vi "PowerRiderDLL_demo.vi"() -> ()   [LabVIEW 2017]
uses:
  Fuse25A_Labview/Power-Rider-GUI/CANalystII/PCAN_Driver/ControlCAN.llb/CAN Channel.ctl
  D:/Projects/GUI/Power Rider Wrapper/PowerRiderDLLWrapper.dll
  PowerRiderDLLWrapper.dll
  Fuse25A_Labview/Power-Rider-GUI/CANalystII/PCAN_Driver/ControlCAN.lvlib
panel:
  in  "TripType Enum":T1(ring)
  in  "Status Enum":enum16{"OFF", "ON", "ERROR", "FOREVER OFF"}(ring)
  out "ch_name":string
  out "unit_name":string
  out "sn_l":string
  out "PN ver":string
  out "SW ver":string
  in  "stop Int":bool
  out "RXdata":T2 {"ID" format="%.0x"}
  in  "Clear Dis":bool
  in  "stop m":bool
  out "String":string
  in  "Tab Control":T3(tab)
  in  "Send":bool
  in  "commandID":u32(ring)=33 items=["ChannelStatus_1"=0, "ChannelControl"=2, "Current_CH1_4"=3, "Current_CH5_8"=4, "Current_CH9_12"=5, "Current_CH13_16"=6, "GetVinVout"=8, "Version_BoardType"=9, "SystemTemp"=10, "SystemParameter"=11, "ChannelParameter"=12, "GetTripEvent"=15, "LogFile"=18, "Configuration"=19, "ProductionData"=20, "BIT"=33, "DiscretePorts"=34, "SerialNumber"=36, "OffsetMeasurement"=37, "PartNumber"=39, "ChannelCombinedStatus_1_CH1_8"=40, "ChannelCombinedStatus_2_CH9_12"=41, "PlotData"=45, "PlotCommand"=46, "InternalData"=47, "KeepAlive"=234, "WakeUp"=250]
  in  "systemParamNumber":u8(ring) items=["SystemUpTime", "UnitIDAddress", "R_Sense", "OpAmpGain", "RingCancelDelay", "VinLowThreshold", "VinHighThresholdP1", "TempLowThreshold", "TempHighThreshold", "GeneralString", "StatusMessage", "SysTime", "CAN_Bitrate", "SerialBaudrate", "DigOutDelayBeforeActive", "DigOutDelayBeforeDeactive", "DigOutOffTimeout", "DigOutControlLow", "DigOutLogicInverse", "DigInputType", "OutputStartupState", "PilotLED_FullScale", "UnitSubAddress", "DigOutControlHigh", "HostAddress", "LogFileDataTime", "OverVoltageTimeP1", "OverVoltageTimeP2", "OverVoltageTimeP3", "VinHighThresholdP2", "VinHighThresholdP3", "TotalUnitCurrentConsumptionScene1", "ChannelPrioritySceneNum", "InputFunctionMode", "InputLogicInverse", "TotalUnitCurrentConsumptionScene2", "TotalUnitCurrentConsumptionScene3", "OverVoltageVin1RetryDelay", "OverVoltageVin2RetryDelay", "VoltageLowHysteresis", "VoltageHighHysteresis", "CommunicationTimeout", "DigitalInputConfig"]
  in  "Sys Param":bool
  in  "CHParamNumber":u8(ring) items=["OverloadThreshold"=0, "Zone2Delay"=1, "HardShortRetryDelay"=2, "HardShortNumOfRetries"=3, "ActiveOnStartup"=4, "GeneralString"=5, "ChCommunicationControl"=6, "SW_TrippedRetryDelay"=7, "SW_TrippedNumOfRetries"=8, "ChStatusResetDelay"=9, "OverloadTime"=10, "I_MaxZone3Time"=11, "I_MaxZone3Threshold"=12, "NominalCurrentValue"=13, "I_2tThreshold"=14, "GroupChannelControl"=15, "TechData"=16, "PWM_Frequency"=17, "PWM_DutyCycle"=18, "PowerProtection"=19, "I_MaxZone2Threshold"=20, "PWM_Control"=21, "ChDelayBeforeOpening"=22, "ChDelayBeforeClosing"=23, "ChOffTimeout"=24, "LogicControl1"=25, "LogicControl2"=26, "I_MaxZone2Time"=27, "LogicControl3"=28, "LogicControl4"=29, "LogEventCurrentThreshold"=30, "OvervoltageNumOfRetries"=32, "ChannelPriorityScene1"=33, "ChannelPriorityScene2"=34, "ChannelPriorityScene3"=35, "I_MinThreshold"=36, "LossCommunicationChannelState"=37, "SoftStopPWM_DC"=38]
  in  "CH Param":bool
  in  "CH Cnt":bool
  in  "SW reset":bool
  in  "Get PN":bool
  in  "Get SW ver":bool
  in  "Get CH Current":bool
  in  "Get CH STS":bool
  in  "Get CH Voltage":bool
  in  "Get CH Name":bool
  in  "Get SN":bool
  in  "Get Unit Name":bool
  in  "Com type":enum32{"CAN", "Serial", "UDP"}(tab)
  in  "Baud":u32(ring)=250000 items=["1M"=1000000, "800K"=800000, "500K"=500000, "250K"=250000, "125K"=125000, "100K"=100000, "83.3K"=83300, "50000"=50000, "20K"=20000, "10K"=10000, "5K"=5000]
  in  "Channel #":T4 caption="Channel" items=["Channel 1", "Channel 2"]
  in  "VISA res_in":refnum<visa-resource-name>
  in  "baud rate":u32(ring)=19200 items=["921600"=921600, "460800"=460800, "256000"=256000, "115200"=115200, "57600"=57600, "38400"=38400, "19200"=19200, "14400"=14400, "9600"=9600, "2400"=2400, "1200"=1200]
  in  "address IP":string="192.168.1.50"
  in  "Port":u16=8030
  in  "Select CH #":u8(ring)=1 items=["CH1"=1, "CH2"=2, "CH3"=3, "CH4"=4, "CH5"=5, "CH6"=6, "CH7"=7, "CH8"=8, "CH9"=9, "CH10"=10, "CH11"=11, "CH12"=12, "CH13"=13, "CH14"=14, "CH15"=15, "CH16"=16]
  out "SendOK":bool
  out "path":path
  out "COM":variant
  out "PowerAddress":u8
  out "HostAddress":u8
  out "CommandID":u8 format="%.0x"
  in  "Dst add":u16=16 format="%.0x"
  in  "address":u16=85 format="%.0x"
  in  "Disonnect":bool
  in  "Connect":bool
  out "CommIcon":bool
  in  "COMType":u16(ring)=2 items=["CANalystII"=2, "TCP Client"=3, "TCP Server"=4, "UDP Client"=5, "Serial COM"=6, "CAN Kvaser"=7]
  in  "payload":u8[](array[numeric])
  out "Payload":u8[](array[numeric]) format="%.0x"
  # "Communication"
  # "Commands"
  # "Responds"
  # "ver 0.1.a"
  # "Power Rider"
  # "REDLER TECHNOLOGIES LTD"
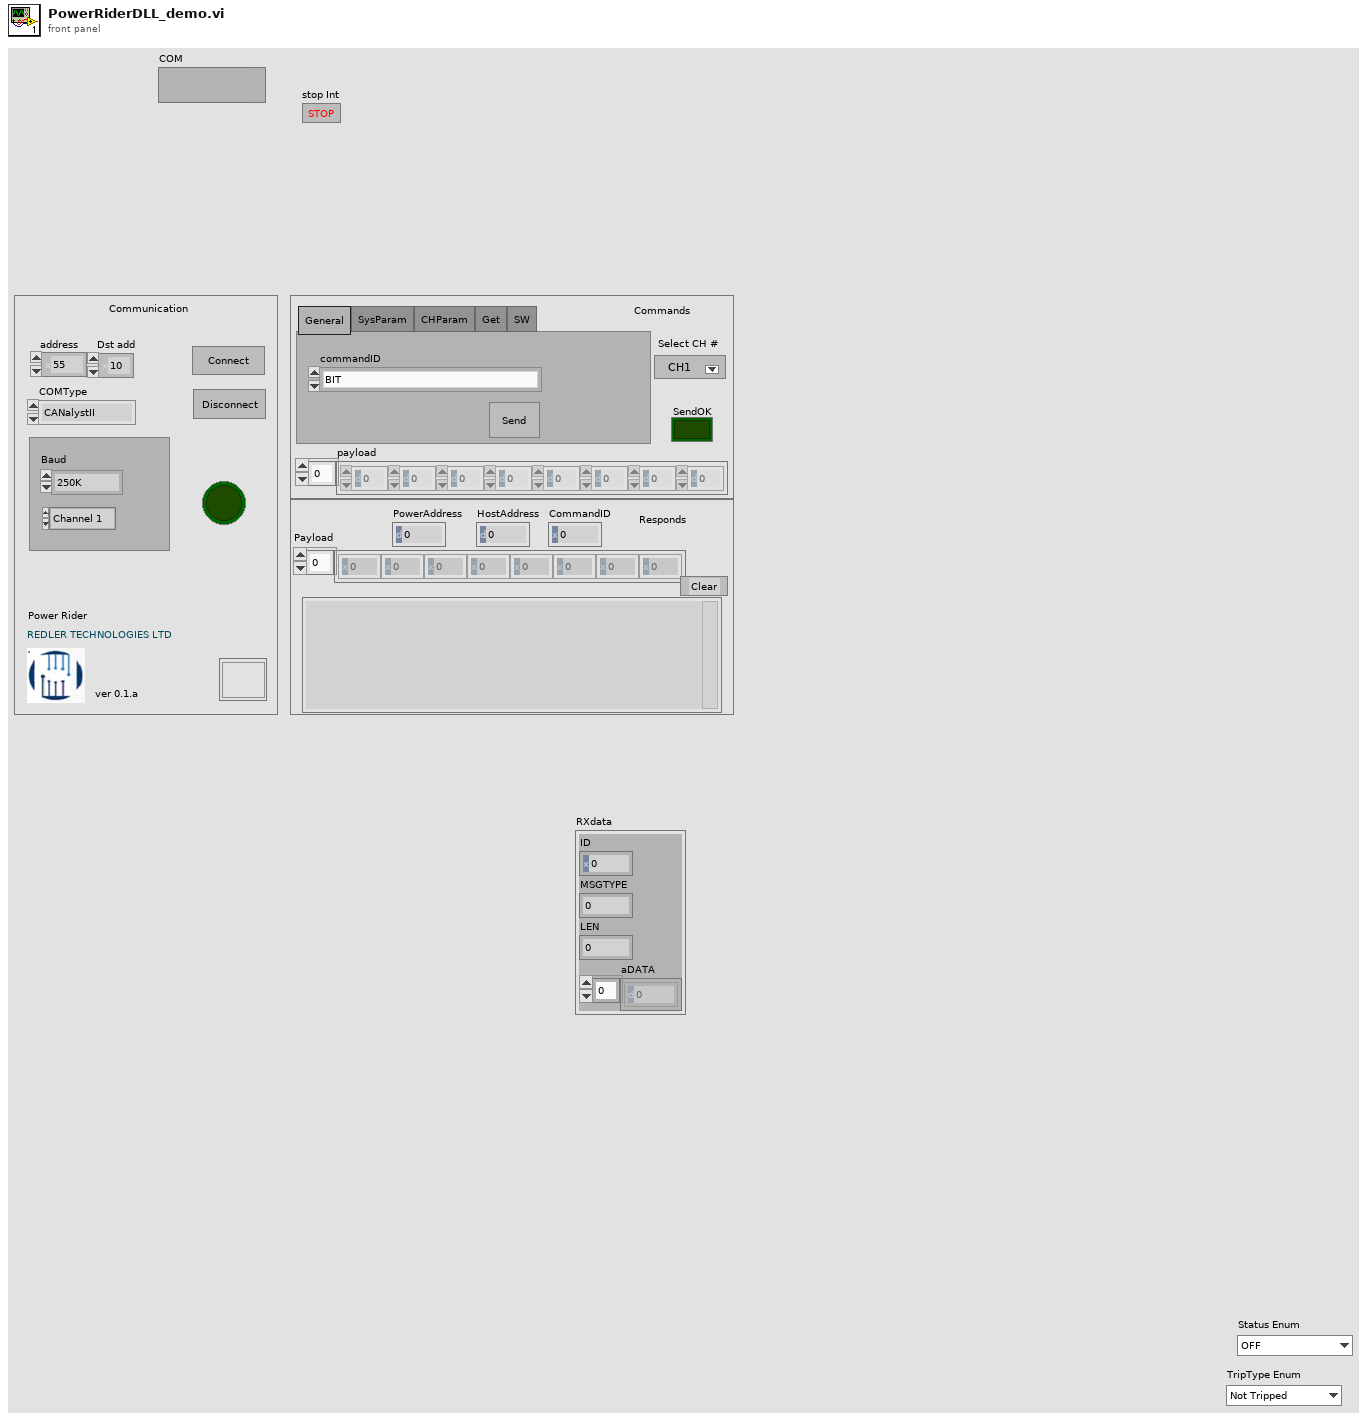
[diagram p1: front panel]
types:
  T1 = enum16{"Not Tripped", "SW Tripped", "Hard Short", "MAX SW Tripped"}
  T2 = cluster{"ID":u32, "MSGTYPE":u8, "LEN":u8, "aDATA":u8[]}
  T3 = enum32{"General", "SysParam", "CHParam", "Get", "SW"}
  T4 = typedef "ControlCAN.lvlib/CAN Channel.ctl" = u32
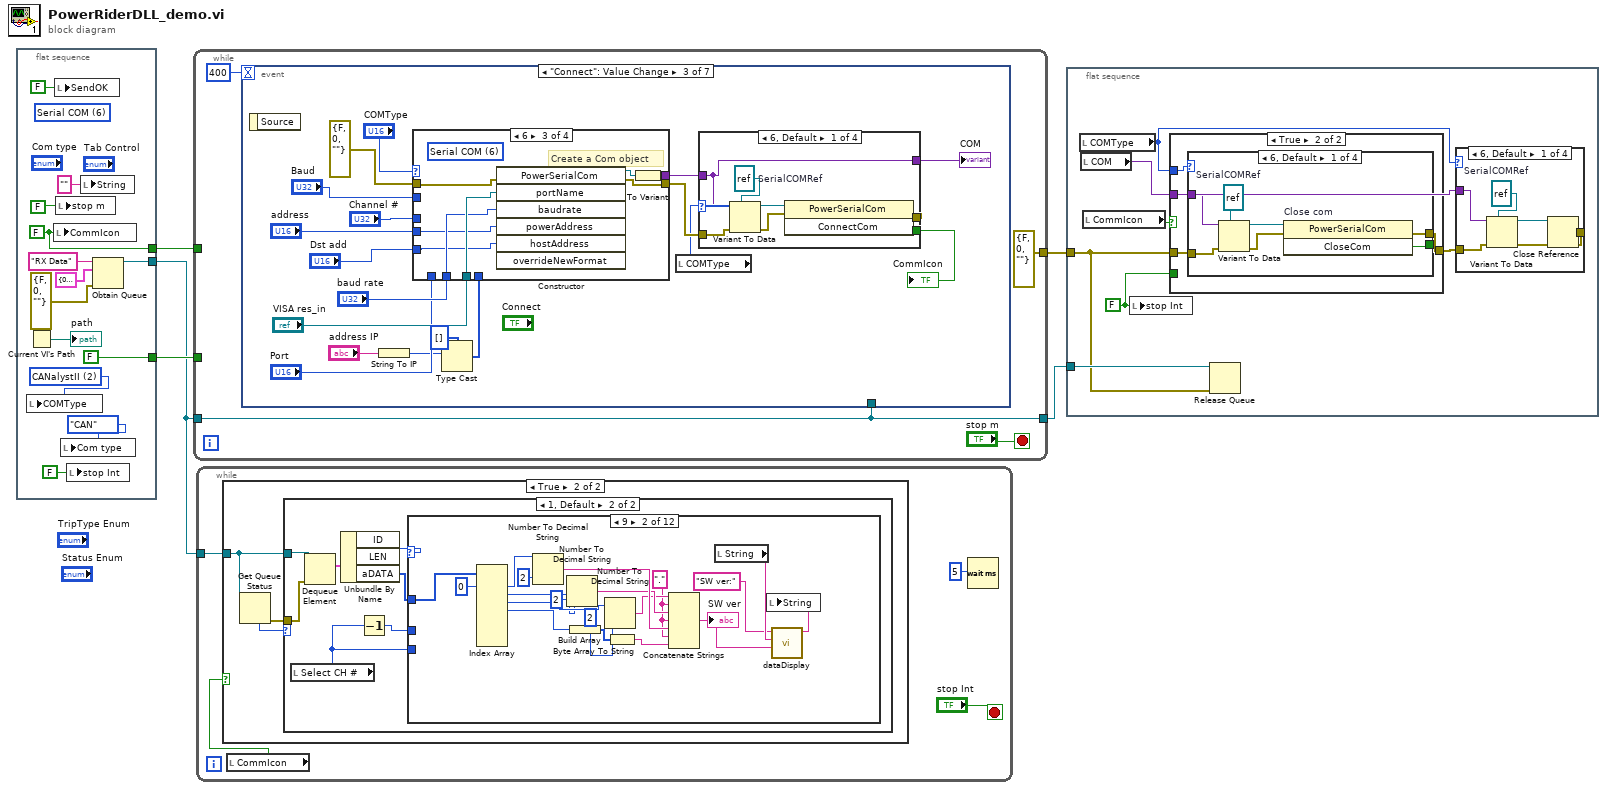
[diagram p0: block diagram]
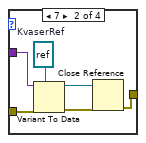
[diagram p2: hidden frame]
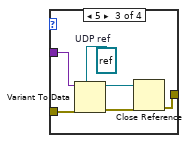
[diagram p3: hidden frame]
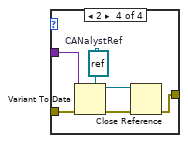
[diagram p4: hidden frame]
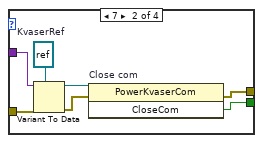
[diagram p6: hidden frame]
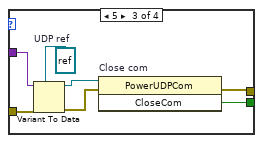
[diagram p7: hidden frame]
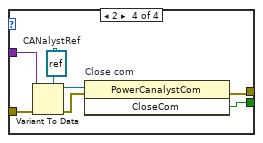
[diagram p8: hidden frame]
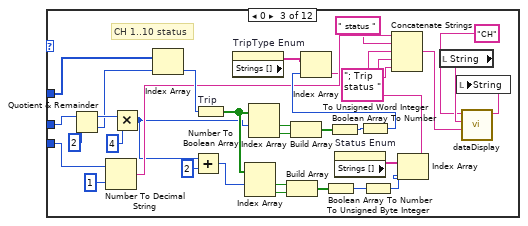
[diagram p12: hidden frame]
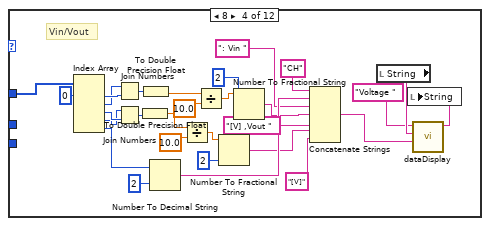
[diagram p13: hidden frame]
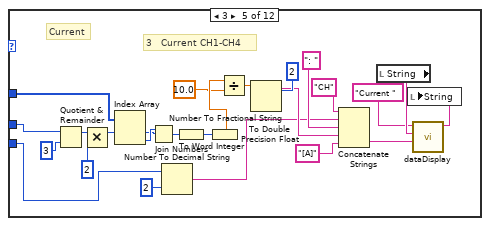
[diagram p14: hidden frame]
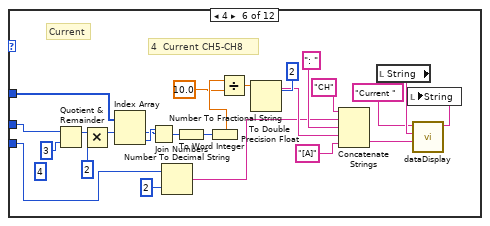
[diagram p15: hidden frame]
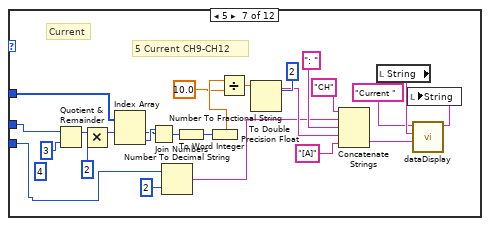
[diagram p16: hidden frame]
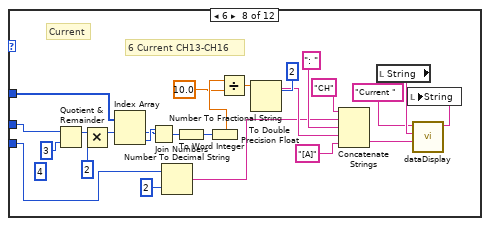
[diagram p17: hidden frame]
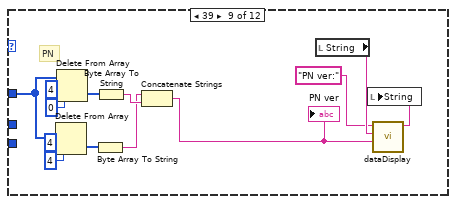
[diagram p18: hidden frame]
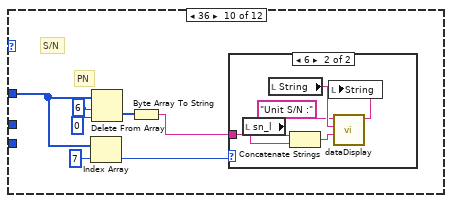
[diagram p19: hidden frame]
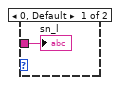
[diagram p20: hidden frame]
diagram:
  n1 = flat-sequence {
    tunnel: [FALSE] -> w4
    tunnel: [w14] -> w3
    tunnel: [w7] -> w2
    frame #0 {
      (unwired) u16 6 items=["CANalystII"=2, "TCP Client"=3, "TCP Server"=4, "UDP Client"=5, "Serial COM"=6, "CAN Kvaser"=7] ("COMType 2")
      w14 = FALSE ("CommIcon")
      w16 = u16 2 items=["CANalystII"=2, "TCP Client"=3, "TCP Server"=4, "UDP Client"=5, "Serial COM"=6, "CAN Kvaser"=7] ("COMType")
      n2 = Current VI's Path() -> (path=→"path":path)
      n3 = local write "COMType"(w16) -> ()
      n4 = local write "CommIcon"(w14) -> ()
      n5 = local write "SendOK"(FALSE ("SendOK")) -> ()
      n6 = local write "stop m"(FALSE ("Exit")) -> ()
      n7 = local write "Com type"(enum32{"CAN", "Serial", "UDP"}."CAN" ("Com type")) -> ()
      n8 = local write "stop Int"(FALSE ("stop Int")) -> ()
      n9 = local write "String"("" ("String")) -> ()
      n10 = Obtain Queue(name (unnamed)="RX Data", element data type=T2 {"ID"=0, "MSGTYPE"=0, "LEN"=0, "aDATA"=[]} ("Msg"), error in (no error)=errorcluster {"status"=FALSE, "code"=0, "source"=""}) -> (queue out=w7:refnum<queue>)  [unwired: 2 in, 2 out]
    }
  }
  n11 = while {
    tunnel: [errorcluster {"status"=FALSE, "code"=0, "source"=""} ("error out")] -> w5
    tunnel: w4 -> [_]
    tunnel: w3 -> [_]
    tunnel: w2 -> [w19]
    tunnel: [w19] -> w1
    stop <- "stop m" stop-if-true
    n12 = event shown="[2] \"Connect\": Value Change" {
      selector: _ -> [_ _ _ _ _ _ _]
      dyn-events: _ -> [_ _ _ _ _ _ _]
      timeout: 400 -> [_ _ _ _ _ _ _]
      tunnel: w19 -> [w23 _ _ _ _ _ _]
      event Timeout {
        n13 = event-data() -> ()  [unwired: 1 in, 1 out]
        n14 = local read "CommIcon"() -> (w24:bool)
        n15 = case shown="True" w24 {
          tunnel: w23 -> [_ w31]
          frame False {
          }
          frame True {
            n16 = local read "COM"() -> (w34:variant)
            n17 = local read "COMType"() -> (w32:u16)
            n18 = case shown="6" w32 {
              selector: w32 -> [w61 w70 w95 w97]
              tunnel: w34 -> [w68 w82 w85 w109]
              tunnel: errorcluster {"status"=FALSE, "code"=0, "source"=""} ("error out") -> [w66 w81 w84 w108]
              tunnel: [w56 w75 w92 w102] -> w29
              tunnel: [w57 w74 w91 w101] -> w30
              tunnel: [w58 w73 w90 w100] -> w28
              tunnel: [w59 w72 w89 w99] -> w27
              tunnel: [w60 w71 w88 w98] -> w26
              tunnel: [w61 w70 w95 w97] -> w25
              tunnel: [w55 w69 w83 w96] -> _
              frame 2, Default {
                w67 = refnum<k24> refnum  # CANalystRef
                n19 = Variant To Data(error in=w66, type=w67, Variant=w68) -> (data=w65:refnum<k24>, error out=w64:errorcluster)
                n20 = invoke class="PowerCanalystCom" method="ReceivePacket"(reference=w65, error in=w64) -> (error out=w62:errorcluster, "ReceivePacket"=w63:refnum<k24>)  [unwired: 1 in, 1 out]
                n21 = property class="PowerPacket"(reference=w63, error in=w62) -> (error out=w55:errorcluster, "CommandID"=w56:u8, "ErrorFlag"=w57:bool, "HostAddress"=w58:u8, "PowerAddress"=w59:u8, "MutablePayload"=w60:u8[])  [unwired: 1 out]
              }
              frame 6 {
                w76 = refnum<k24> refnum  # SerialCOMRef
                n22 = Variant To Data(error in=w81, type=w76, Variant=w82) -> (data=w80:refnum<k24>, error out=w79:errorcluster)
                n23 = invoke class="PowerSerialCom" method="ReceivePacket"(reference=w80, error in=w79) -> (error out=w77:errorcluster, "ReceivePacket"=w78:refnum<k24>)  [unwired: 1 in, 1 out]
                n24 = property class="PowerPacket"(reference=w78, error in=w77) -> (error out=w69:errorcluster, "CommandID"=w75:u8, "ErrorFlag"=w74:bool, "HostAddress"=w73:u8, "PowerAddress"=w72:u8, "MutablePayload"=w71:u8[])  [unwired: 1 out]
              }
              frame 5 {
                w87 = refnum<k24> refnum  # UDP ref
                n25 = Variant To Data(error in=w84, type=w87, Variant=w85) -> (data=w86:refnum<k24>)  [unwired: 1 out]
                n26 = invoke class="PowerUDPCom" method="ReceivePacketAsync"(reference=w86) -> ("ReceivePacketAsync"=w94:refnum<k24>)  [unwired: 2 in, 2 out]
                n27 = property class="Task`1[[PowerRiderDLLWrapper.Po"(reference=w94) -> ("Result"=w93:refnum<k24>)  [unwired: 1 in, 2 out]
                n28 = property class="PowerPacket"(reference=w93) -> (error out=w83:errorcluster, "CommandID"=w92:u8, "ErrorFlag"=w91:bool, "HostAddress"=w90:u8, "PowerAddress"=w89:u8, "MutablePayload"=w88:u8[])  [unwired: 1 in, 1 out]
              }
              frame 7 {
                w103 = refnum<k24> refnum  # KvaserRef
                n29 = Variant To Data(error in=w108, type=w103, Variant=w109) -> (data=w107:refnum<k24>, error out=w106:errorcluster)
                n30 = invoke class="PowerKvaserCom" method="ReceivePacket"(reference=w107, error in=w106) -> (error out=w104:errorcluster, "ReceivePacket"=w105:refnum<k24>)  [unwired: 1 in, 1 out]
                n31 = property class="PowerPacket"(reference=w105, error in=w104) -> (error out=w96:errorcluster, "CommandID"=w102:u8, "ErrorFlag"=w101:bool, "HostAddress"=w100:u8, "PowerAddress"=w99:u8, "MutablePayload"=w98:u8[])  [unwired: 1 out]
              }
            }
            n32 = case shown="False" w30 {
              tunnel: w26 -> [w39 w47]
              tunnel: w27 -> [w45 _]
              tunnel: w28 -> [w46 _]
              tunnel: w29 -> [w40 _]
              tunnel: w25 -> [w38 _]
              tunnel: w31 -> [w36 _]
              frame False {
                # "OK"
                n33 = local read "String"() -> (w43:string)
                n34 = call "StrDisplay.vi"("Payload"=w39, "ID"=w40, "string in"=w43, "string type"="RX") -> ("str out"=→"String":string)  [unwired: 7 in]
                n35 = Bundle By Name(cluster=T2 {"ID"=0, "MSGTYPE"=0, "LEN"=0, "aDATA"=[]} ("Msg"), "ID"=w40, "MSGTYPE"=w38, "LEN"=u8 0, "aDATA"=w39) -> (w35:T2)
                "RXdata" <- w35
                n36 = Enqueue Element(queue=w36, element=w35) -> ()  [unwired: 1 in, 4 out]
                "Payload" <- w39
                "CommandID" <- w40
                "HostAddress" <- w46
                "PowerAddress" <- w45
              }
              frame True {
                n37 = Index Array(array=w47, index=0) -> (element=w48:u8)
                n38 = case shown="1, Default" w48 {
                  tunnel: w48 -> [_ w54]
                  tunnel: w47 -> [_ _]
                  frame 9 {
                  }
                  frame 1, Default {
                    # "Error"
                    n39 = Number To Decimal String(number=w54) -> (decimal integer string=w50:string)  [unwired: 1 in]
                    n40 = local read "String"() -> (w52:string)
                    n41 = call "StrDisplay.vi"("Err str"=w50, "string in"=w52, "string type"="Error") -> ("str out"=w53:string)  [unwired: 8 in]
                    n42 = local write "String"(w53) -> ()
                  }
                }
              }
            }
          }
        }
      }
      event "Clear Dis": Value Change {
        n43 = event-data() -> ()  [unwired: 1 in, 6 out]
        n44 = local write "String"("" ("String")) -> ()
      }
      event "Connect": Value Change {
        n45 = event-data() -> ()  [unwired: 1 in, 1 out]
        n46 = String To IP(1:"address IP") -> (0:w113:u32)
        n47 = Type Cast(type=u8[] [] ("powerIPAddress"), x=w113) -> (*(type *) &x=w111:u8[])
        n48 = case shown="6" "COMType" {
          tunnel: [w164 w172 w180 w188] -> w125
          tunnel: [w157 w166 w178 w186] -> w126
          tunnel: "Baud" -> [w162 w170 _ _]
          tunnel: "Dst add" -> [w159 w167 w173 w181]
          tunnel: "address" -> [w160 w168 w174 w182]
          tunnel: "Channel #" -> [w161 w169 _ _]
          tunnel: errorcluster {"status"=FALSE, "code"=0, "source"=""} ("error out") -> [w163 w171 w177 w185]
          tunnel: "baud rate" -> [_ _ w175 _]
          tunnel: "VISA res_in" -> [_ _ w176 _]
          tunnel: "Port" -> [_ _ _ w183]
          tunnel: w111 -> [_ _ _ w184]
          frame 2, Default {
            (unwired) u16 2 items=["CANalystII"=2, "TCP Client"=3, "TCP Server"=4, "UDP Client"=5, "Serial COM"=6, "CAN Kvaser"=7] ("COMType 2")
            n49 = constructor class="PowerCanalystCom"(error in=w163, "bitrate"=w162, "deviceIndex"=w161, "powerAddress"=w160, "hostAddress"=w159) -> (reference out=w158:refnum<k24>, error out=w157:errorcluster)  [unwired: 2 in, 5 out]
            n50 = To Variant(anything=w158) -> (Variant=w164:variant)
          }
          frame 7 {
            (unwired) u16 7 items=["CANalystII"=2, "TCP Client"=3, "TCP Server"=4, "UDP Client"=5, "Serial COM"=6, "CAN Kvaser"=7] ("COMType 2")
            n51 = constructor class="PowerKvaserCom"(error in=w171, "bitrate"=w170, "deviceIndex"=w169, "powerAddress"=w168, "hostAddress"=w167) -> (reference out=w165:refnum<k24>, error out=w166:errorcluster)  [unwired: 2 in, 5 out]
            n52 = To Variant(anything=w165) -> (Variant=w172:variant)
          }
          frame 6 {
            (unwired) u16 6 items=["CANalystII"=2, "TCP Client"=3, "TCP Server"=4, "UDP Client"=5, "Serial COM"=6, "CAN Kvaser"=7] ("COMType 2")
            # "Create a Com object"
            n53 = constructor class="PowerSerialCom"(error in=w177, "portName"=w176, "baudrate"=w175, "powerAddress"=w174, "hostAddress"=w173) -> (reference out=w179:refnum<k24>, error out=w178:errorcluster)  [unwired: 3 in, 6 out]
            n54 = To Variant(anything=w179) -> (Variant=w180:variant)
          }
          frame 5 {
            (unwired) u16 5 items=["CANalystII"=2, "TCP Client"=3, "TCP Server"=4, "UDP Client"=5, "Serial COM"=6, "CAN Kvaser"=7] ("COMType 2")
            n55 = constructor class="PowerUDPCom"(error in=w185, "powerIPAddress"=w184, "powerPort"=w183, "powerAddress"=w182, "hostAddress"=w181) -> (reference out=w187:refnum<k24>, error out=w186:errorcluster)  [unwired: 2 in, 5 out]
            n56 = To Variant(anything=w187) -> (Variant=w188:variant)
          }
        }
        n57 = local read "COMType"() -> (w124:u16)
        n58 = case shown="6, Default" w124 {
          tunnel: w125 -> [w129 w136 w143 w151]
          tunnel: [w131 w137 w146 w154] -> w128
          tunnel: w126 -> [w135 w142 w145 w153]
          tunnel: [w130 w138 w144 w152] -> _
          tunnel: [w129 w136 w143 w151] -> w116
          frame 6, Default {
            w134 = refnum<k24> refnum  # SerialCOMRef
            n59 = Variant To Data(error in=w135, type=w134, Variant=w129) -> (data=w133:refnum<k24>, error out=w132:errorcluster)
            n60 = invoke class="PowerSerialCom" method="ConnectCom"(reference=w133, error in=w132) -> (error out=w130:errorcluster, "ConnectCom"=w131:bool)  [unwired: 1 in, 1 out]
          }
          frame 7 {
            w139 = refnum<k24> refnum  # KvaserRef
            n61 = Variant To Data(error in=w142, type=w139, Variant=w136) -> (data=w140:refnum<k24>, error out=w141:errorcluster)
            n62 = invoke class="PowerKvaserCom" method="ConnectCom"(reference=w140, error in=w141) -> (error out=w138:errorcluster, "ConnectCom"=w137:bool)  [unwired: 1 in, 1 out]
          }
          frame 2 {
            w149 = refnum<k24> refnum  # CANalystRef
            n63 = Variant To Data(error in=w145, type=w149, Variant=w143) -> (data=w148:refnum<k24>, error out=w147:errorcluster)
            n64 = invoke class="PowerCanalystCom" method="ConnectCom"(reference=w148, error in=w147) -> (error out=w144:errorcluster, "ConnectCom"=w146:bool)  [unwired: 1 in, 1 out]
          }
          frame 5 {
            w150 = refnum<k24> refnum  # UDP ref
            n65 = Variant To Data(error in=w153, type=w150, Variant=w151) -> (data=w156:refnum<k24>, error out=w155:errorcluster)
            n66 = invoke class="PowerUDPCom" method="ConnectCom"(reference=w156, error in=w155) -> (error out=w152:errorcluster, "ConnectCom"=w154:bool)  [unwired: 1 in, 1 out]
          }
        }
        "CommIcon" <- w128
        "COM" <- w116
      }
      event "Get SW ver", "Get CH Voltage", "Get CH STS", "Get CH Current", "Get PN", "SW reset", "Get SN", "Get CH Name", "Get Unit Name", "CH Cnt": Value Change {
        w189 = FALSE ("SendOK")
        n67 = event-data() -> ("CtlRef"=w192:refnum<vi>)  [unwired: 1 in]
        n68 = local write "SendOK"(w189) -> ()
        n69 = local read "CommIcon"() -> (w198:bool)
        n70 = property class="Bool"(reference=w192) -> ("Label.Text"=w191:string)  [unwired: 1 in, 2 out]
        n71 = local read "COM"() -> (w199:variant)
        n72 = local read "COMType"() -> (w200:u16)
        n73 = case shown="True" w198 {
          tunnel: w200 -> [_ w210]
          tunnel: u8 6 ("priority") -> [_ w209]
          tunnel: "commandID" -> [_ w208]
          tunnel: "payload" -> [_ w207]
          tunnel: w199 -> [_ w206]
          tunnel: errorcluster {"status"=FALSE, "code"=0, "source"=""} ("error out") -> [_ w205]
          tunnel: [FALSE ("SendPacket") w204] -> w193
          tunnel: w191 -> [_ w203]
          tunnel: "Select CH #" -> [_ w202]
          tunnel: w189 -> [_ _]
          frame False {
          }
          frame True {
            n74 = case shown="6, Default" w210 {
              tunnel: w206 -> [w222 w350 w478 w606]
              tunnel: [w211 w339 w473 w601] -> w204
              tunnel: w205 -> [w221 w349 w476 w605]
              tunnel: [w212 w347 w474 w602] -> _
              tunnel: w209 -> [w216 w343 w471 w600]
              tunnel: w208 -> [w215 w342 w470 w599]
              tunnel: w207 -> [w214 w341 w469 w598]
              tunnel: w203 -> [w219 w346 w467 w603]
              tunnel: w202 -> [w213 w340 w468 w597]
              frame 6, Default {
                w220 = refnum<k24> refnum  # SerialCOMRef
                n75 = Variant To Data(error in=w221, type=w220, Variant=w222) -> (data=w217:refnum<k24>, error out=w218:errorcluster)
                n76 = case shown="\"Get SW ver\"" w219 {
                  tunnel: w218 -> [w229 w236 w243 w250 w257 w265 w277 w303 w306 w312 w317 w329 w336]
                  tunnel: [w228 w235 w242 w249 w256 w264 w276 w302 w308 w315 w321 w332 w335] -> w212
                  tunnel: [w227 w234 w241 w248 w255 w263 w275 w301 w309 w314 w324 w331 w334] -> w211
                  tunnel: w217 -> [w226 w233 w240 w247 w254 w262 w274 w300 w307 w313 w318 w330 w337]
                  tunnel: w216 -> [w225 w232 w239 w246 w253 w261 w273 w299 w305 w311 w323 w328 w338]
                  tunnel: w215 -> [w224 _ _ _ _ _ _ _ _ _ _ _ _]
                  tunnel: w214 -> [w223 w231 w238 w245 w252 w260 _ _ _ _ w320 w326 _]
                  tunnel: w213 -> [_ _ _ _ _ w258 w271 w287 _ _ w322 _ w333]
                  frame "Send", Default {
                    n77 = invoke class="PowerSerialCom" method="SendPacket"(reference=w226, error in=w229, "priority"=w225, "commandID"=w224, "payload"=w223) -> (error out=w228:errorcluster, "SendPacket"=w227:bool)  [unwired: 1 in, 4 out]
                  }
                  frame "Get SW ver" {
                    w230 = u8 9 items=["ChannelStatus_1"=0, "ChannelControl"=2, "Current_CH1_4"=3, "Current_CH5_8"=4, "Current_CH9_12"=5, "Current_CH13_16"=6, "GetVinVout"=8, "Version_BoardType"=9, "SystemTemp"=10, "SystemParameter"=11, "ChannelParameter"=12, "GetTripEvent"=15, "LogFile"=18, "Configuration"=19, "ProductionData"=20, "BIT"=33, "DiscretePorts"=34, "SerialNumber"=36, "OffsetMeasurement"=37, "PartNumber"=39, "ChannelCombinedStatus_1_CH1_8"=40, "ChannelCombinedStatus_2_CH9_12"=41, "PlotData"=45, "PlotCommand"=46, "InternalData"=47, "KeepAlive"=234, "WakeUp"=250] ("commandID")
                    n78 = invoke class="PowerSerialCom" method="SendPacket"(reference=w233, error in=w236, "priority"=w232, "commandID"=w230, "payload"=w231) -> (error out=w235:errorcluster, "SendPacket"=w234:bool)  [unwired: 1 in, 4 out]
                  }
                  frame "Get PN" {
                    w237 = u8 39 items=["ChannelStatus_1"=0, "ChannelControl"=2, "Current_CH1_4"=3, "Current_CH5_8"=4, "Current_CH9_12"=5, "Current_CH13_16"=6, "GetVinVout"=8, "Version_BoardType"=9, "SystemTemp"=10, "SystemParameter"=11, "ChannelParameter"=12, "GetTripEvent"=15, "LogFile"=18, "Configuration"=19, "ProductionData"=20, "BIT"=33, "DiscretePorts"=34, "SerialNumber"=36, "OffsetMeasurement"=37, "PartNumber"=39, "ChannelCombinedStatus_1_CH1_8"=40, "ChannelCombinedStatus_2_CH9_12"=41, "PlotData"=45, "PlotCommand"=46, "InternalData"=47, "KeepAlive"=234, "WakeUp"=250] ("commandID")
                    n79 = invoke class="PowerSerialCom" method="SendPacket"(reference=w240, error in=w243, "priority"=w239, "commandID"=w237, "payload"=w238) -> (error out=w242:errorcluster, "SendPacket"=w241:bool)  [unwired: 1 in, 4 out]
                  }
                  frame "SW reset" {
                    w244 = u8 36 items=["ChannelStatus_1"=0, "ChannelControl"=2, "Current_CH1_4"=3, "Current_CH5_8"=4, "Current_CH9_12"=5, "Current_CH13_16"=6, "GetVinVout"=8, "Version_BoardType"=9, "SystemTemp"=10, "SystemParameter"=11, "ChannelParameter"=12, "GetTripEvent"=15, "LogFile"=18, "Configuration"=19, "ProductionData"=20, "BIT"=33, "DiscretePorts"=34, "SerialNumber"=36, "OffsetMeasurement"=37, "PartNumber"=39, "ChannelCombinedStatus_1_CH1_8"=40, "ChannelCombinedStatus_2_CH9_12"=41, "PlotData"=45, "PlotCommand"=46, "InternalData"=47, "KeepAlive"=234, "WakeUp"=250] ("commandID")
                    n80 = invoke class="PowerSerialCom" method="SendPacket"(reference=w247, error in=w250, "priority"=w246, "commandID"=w244, "payload"=w245) -> (error out=w249:errorcluster, "SendPacket"=w248:bool)  [unwired: 1 in, 4 out]
                  }
                  frame "Get CH STS" {
                    w251 = u8 0 items=["ChannelStatus_1"=0, "ChannelControl"=2, "Current_CH1_4"=3, "Current_CH5_8"=4, "Current_CH9_12"=5, "Current_CH13_16"=6, "GetVinVout"=8, "Version_BoardType"=9, "SystemTemp"=10, "SystemParameter"=11, "ChannelParameter"=12, "GetTripEvent"=15, "LogFile"=18, "Configuration"=19, "ProductionData"=20, "BIT"=33, "DiscretePorts"=34, "SerialNumber"=36, "OffsetMeasurement"=37, "PartNumber"=39, "ChannelCombinedStatus_1_CH1_8"=40, "ChannelCombinedStatus_2_CH9_12"=41, "PlotData"=45, "PlotCommand"=46, "InternalData"=47, "KeepAlive"=234, "WakeUp"=250] ("commandID")
                    n81 = invoke class="PowerSerialCom" method="SendPacket"(reference=w254, error in=w257, "priority"=w253, "commandID"=w251, "payload"=w252) -> (error out=w256:errorcluster, "SendPacket"=w255:bool)  [unwired: 1 in, 4 out]
                  }
                  frame "Get CH Current" {
                    n82 = case shown="1..4, Default" w258 {
                      tunnel: [w266 w267 w268 w269] -> w259
                      frame 1..4, Default {
                        w266 = u8 3 items=["ChannelStatus_1"=0, "ChannelControl"=2, "Current_CH1_4"=3, "Current_CH5_8"=4, "Current_CH9_12"=5, "Current_CH13_16"=6, "GetVinVout"=8, "Version_BoardType"=9, "SystemTemp"=10, "SystemParameter"=11, "ChannelParameter"=12, "GetTripEvent"=15, "LogFile"=18, "Configuration"=19, "ProductionData"=20, "BIT"=33, "DiscretePorts"=34, "SerialNumber"=36, "OffsetMeasurement"=37, "PartNumber"=39, "ChannelCombinedStatus_1_CH1_8"=40, "ChannelCombinedStatus_2_CH9_12"=41, "PlotData"=45, "PlotCommand"=46, "InternalData"=47, "KeepAlive"=234, "WakeUp"=250] ("commandID")
                      }
                      frame 5..8 {
                        w267 = u8 4 items=["ChannelStatus_1"=0, "ChannelControl"=2, "Current_CH1_4"=3, "Current_CH5_8"=4, "Current_CH9_12"=5, "Current_CH13_16"=6, "GetVinVout"=8, "Version_BoardType"=9, "SystemTemp"=10, "SystemParameter"=11, "ChannelParameter"=12, "GetTripEvent"=15, "LogFile"=18, "Configuration"=19, "ProductionData"=20, "BIT"=33, "DiscretePorts"=34, "SerialNumber"=36, "OffsetMeasurement"=37, "PartNumber"=39, "ChannelCombinedStatus_1_CH1_8"=40, "ChannelCombinedStatus_2_CH9_12"=41, "PlotData"=45, "PlotCommand"=46, "InternalData"=47, "KeepAlive"=234, "WakeUp"=250] ("commandID")
                      }
                      frame 9..12 {
                        w268 = u8 5 items=["ChannelStatus_1"=0, "ChannelControl"=2, "Current_CH1_4"=3, "Current_CH5_8"=4, "Current_CH9_12"=5, "Current_CH13_16"=6, "GetVinVout"=8, "Version_BoardType"=9, "SystemTemp"=10, "SystemParameter"=11, "ChannelParameter"=12, "GetTripEvent"=15, "LogFile"=18, "Configuration"=19, "ProductionData"=20, "BIT"=33, "DiscretePorts"=34, "SerialNumber"=36, "OffsetMeasurement"=37, "PartNumber"=39, "ChannelCombinedStatus_1_CH1_8"=40, "ChannelCombinedStatus_2_CH9_12"=41, "PlotData"=45, "PlotCommand"=46, "InternalData"=47, "KeepAlive"=234, "WakeUp"=250] ("commandID")
                      }
                      frame 13..16 {
                        w269 = u8 6 items=["ChannelStatus_1"=0, "ChannelControl"=2, "Current_CH1_4"=3, "Current_CH5_8"=4, "Current_CH9_12"=5, "Current_CH13_16"=6, "GetVinVout"=8, "Version_BoardType"=9, "SystemTemp"=10, "SystemParameter"=11, "ChannelParameter"=12, "GetTripEvent"=15, "LogFile"=18, "Configuration"=19, "ProductionData"=20, "BIT"=33, "DiscretePorts"=34, "SerialNumber"=36, "OffsetMeasurement"=37, "PartNumber"=39, "ChannelCombinedStatus_1_CH1_8"=40, "ChannelCombinedStatus_2_CH9_12"=41, "PlotData"=45, "PlotCommand"=46, "InternalData"=47, "KeepAlive"=234, "WakeUp"=250] ("commandID")
                      }
                    }
                    n83 = invoke class="PowerSerialCom" method="SendPacket"(reference=w262, error in=w265, "priority"=w261, "commandID"=w259, "payload"=w260) -> (error out=w264:errorcluster, "SendPacket"=w263:bool)  [unwired: 1 in, 4 out]
                  }
                  frame "Get CH Voltage" {
                    w272 = u8 8 items=["ChannelStatus_1"=0, "ChannelControl"=2, "Current_CH1_4"=3, "Current_CH5_8"=4, "Current_CH9_12"=5, "Current_CH13_16"=6, "GetVinVout"=8, "Version_BoardType"=9, "SystemTemp"=10, "SystemParameter"=11, "ChannelParameter"=12, "GetTripEvent"=15, "LogFile"=18, "Configuration"=19, "ProductionData"=20, "BIT"=33, "DiscretePorts"=34, "SerialNumber"=36, "OffsetMeasurement"=37, "PartNumber"=39, "ChannelCombinedStatus_1_CH1_8"=40, "ChannelCombinedStatus_2_CH9_12"=41, "PlotData"=45, "PlotCommand"=46, "InternalData"=47, "KeepAlive"=234, "WakeUp"=250] ("commandID")
                    n84 = Build Array(w271) -> (w270:u8[])
                    n85 = invoke class="PowerSerialCom" method="SendPacket"(reference=w274, error in=w277, "priority"=w273, "commandID"=w272, "payload"=w270) -> (error out=w276:errorcluster, "SendPacket"=w275:bool)  [unwired: 1 in, 4 out]
                  }
                  frame "CH Cnt" {
                    w298 = u8 2 items=["ChannelStatus_1"=0, "ChannelControl"=2, "Current_CH1_4"=3, "Current_CH5_8"=4, "Current_CH9_12"=5, "Current_CH13_16"=6, "GetVinVout"=8, "Version_BoardType"=9, "SystemTemp"=10, "SystemParameter"=11, "ChannelParameter"=12, "GetTripEvent"=15, "LogFile"=18, "Configuration"=19, "ProductionData"=20, "BIT"=33, "DiscretePorts"=34, "SerialNumber"=36, "OffsetMeasurement"=37, "PartNumber"=39, "ChannelCombinedStatus_1_CH1_8"=40, "ChannelCombinedStatus_2_CH9_12"=41, "PlotData"=45, "PlotCommand"=46, "InternalData"=47, "KeepAlive"=234, "WakeUp"=250] ("commandID")
                    n86 = Decrement(x=w287) -> (x-1=w297:u8)
                    n87 = local read "CH Cnt"() -> (w278:bool)
                    n88 = To Long Integer(number=w297) -> (32bit integer=w291:i32)
                    n89 = Number To Boolean Array(number=u16 0 ("element")) -> (Boolean array=w295:bool[])
                    n90 = Replace Array Subset(array=w295, new element=w278, index=w291) -> (w294:bool[])
                    n91 = Number To Boolean Array(number=u16 4095 ("mask")) -> (Boolean array=w292:bool[])
                    n92 = Boolean Array To Number(Boolean array=w294) -> (number=w293:u32)
                    n93 = To Unsigned Word Integer(number=w293) -> (unsigned 16bit integer=w285:u16)
                    n94 = Replace Array Subset(array=w292, new element=FALSE ("new element/subarray"), index=w291) -> (w296:bool[])
                    n95 = Split Number(x=w285) -> (hi(x)=w281:u8, lo(x)=w282:u8)
                    n96 = Boolean Array To Number(Boolean array=w296) -> (number=w286:u32)
                    n97 = To Unsigned Word Integer(number=w286) -> (unsigned 16bit integer=w283:u16)
                    n98 = Split Number(x=w283) -> (hi(x)=w279:u8, lo(x)=w280:u8)
                    n99 = Build Array(w282, w280, w281, w279) -> (w284:u8[])
                    n100 = invoke class="PowerSerialCom" method="SendPacket"(reference=w300, error in=w303, "priority"=w299, "commandID"=w298, "payload"=w284) -> (error out=w302:errorcluster, "SendPacket"=w301:bool)  [unwired: 1 in, 4 out]
                  }
                  frame "Get Unit Name" {
                    n101 = invoke on="Unit name 8msg" class="PowerSerialCom" method="AskSysUnitName"(reference=w307, error in=w306, "priority"=w305) -> (error out=w308:errorcluster, "AskSysUnitName"=w309:bool)  [unwired: 1 in, 2 out]
                    n102 = local write "unit_name"("" ("unit_name")) -> ()
                  }
                  frame "Get SN" {
                    n103 = invoke on="S/n 2msg" class="PowerSerialCom" method="AskSerialNumber"(reference=w313, error in=w312, "priority"=w311) -> (error out=w315:errorcluster, "AskSerialNumber"=w314:bool)  [unwired: 1 in, 2 out]
                    n104 = local write "sn_l"("" ("sn_l")) -> ()
                  }
                  frame "CH Param" {
                    n105 = local read "CHParamNumber"() -> (w316:u8)
                    n106 = Array Size(array=w320) -> (size(s)=w319:i32)
                    n107 = invoke on="CH param" class="PowerSerialCom" method="SendChannelParamPacket"(reference=w318, error in=w317, "priority"=w323, "systemParamNumber"=w316, "channelNum"=w322, "payload"=w320, "strInd"=w319) -> (error out=w321:errorcluster, "SendChannelParamPacket"=w324:bool)  [unwired: 1 in, 6 out]
                  }
                  frame "Sys Param" {
                    n108 = local read "systemParamNumber"() -> (w325:u8)
                    n109 = Array Size(array=w326) -> (size(s)=w327:i32)
                    n110 = invoke on="Sys param" class="PowerSerialCom" method="SendSysParamPacket"(reference=w330, error in=w329, "priority"=w328, "systemParamNumber"=w325, "payload"=w326, "strInd"=w327) -> (error out=w332:errorcluster, "SendSysParamPacket"=w331:bool)  [unwired: 1 in, 5 out]
                  }
                  frame "Get CH Name" {
                    n111 = invoke on="CH name , 6cmd" class="PowerSerialCom" method="AskChannelUnitName"(reference=w337, error in=w336, "priority"=w338, "channelNumber"=w333) -> (error out=w335:errorcluster, "AskChannelUnitName"=w334:bool)  [unwired: 1 in, 3 out]
                  }
                }
              }
              frame 7 {
                w348 = refnum<k24> refnum  # KvaserRef
                n112 = Variant To Data(error in=w349, type=w348, Variant=w350) -> (data=w345:refnum<k24>, error out=w344:errorcluster)
                n113 = case shown="\"Get SW ver\"" w346 {
                  tunnel: w344 -> [w357 w364 w371 w378 w385 w393 w405 w431 w434 w440 w445 w457 w464]
                  tunnel: [w356 w363 w370 w377 w384 w392 w404 w430 w436 w443 w449 w460 w463] -> w347
                  tunnel: [w355 w362 w369 w376 w383 w391 w403 w429 w437 w442 w452 w459 w462] -> w339
                  tunnel: w345 -> [w354 w361 w368 w375 w382 w390 w402 w428 w435 w441 w446 w458 w465]
                  tunnel: w343 -> [w353 w360 w367 w374 w381 w389 w401 w427 w433 w439 w451 w456 w466]
                  tunnel: w342 -> [w352 _ _ _ _ _ _ _ _ _ _ _ _]
                  tunnel: w341 -> [w351 w359 w366 w373 w380 w388 _ _ _ _ w448 w454 _]
                  tunnel: w340 -> [_ _ _ _ _ w386 w399 w415 _ _ w450 _ w461]
                  frame "Send", Default {
                    n114 = invoke class="PowerKvaserCom" method="SendPacket"(reference=w354, error in=w357, "priority"=w353, "commandID"=w352, "payload"=w351) -> (error out=w356:errorcluster, "SendPacket"=w355:bool)  [unwired: 1 in, 4 out]
                  }
                  frame "Get SW ver" {
                    w358 = u8 9 items=["ChannelStatus_1"=0, "ChannelControl"=2, "Current_CH1_4"=3, "Current_CH5_8"=4, "Current_CH9_12"=5, "Current_CH13_16"=6, "GetVinVout"=8, "Version_BoardType"=9, "SystemTemp"=10, "SystemParameter"=11, "ChannelParameter"=12, "GetTripEvent"=15, "LogFile"=18, "Configuration"=19, "ProductionData"=20, "BIT"=33, "DiscretePorts"=34, "SerialNumber"=36, "OffsetMeasurement"=37, "PartNumber"=39, "ChannelCombinedStatus_1_CH1_8"=40, "ChannelCombinedStatus_2_CH9_12"=41, "PlotData"=45, "PlotCommand"=46, "InternalData"=47, "KeepAlive"=234, "WakeUp"=250] ("commandID")
                    n115 = invoke class="PowerKvaserCom" method="SendPacket"(reference=w361, error in=w364, "priority"=w360, "commandID"=w358, "payload"=w359) -> (error out=w363:errorcluster, "SendPacket"=w362:bool)  [unwired: 1 in, 4 out]
                  }
                  frame "Get PN" {
                    w365 = u8 39 items=["ChannelStatus_1"=0, "ChannelControl"=2, "Current_CH1_4"=3, "Current_CH5_8"=4, "Current_CH9_12"=5, "Current_CH13_16"=6, "GetVinVout"=8, "Version_BoardType"=9, "SystemTemp"=10, "SystemParameter"=11, "ChannelParameter"=12, "GetTripEvent"=15, "LogFile"=18, "Configuration"=19, "ProductionData"=20, "BIT"=33, "DiscretePorts"=34, "SerialNumber"=36, "OffsetMeasurement"=37, "PartNumber"=39, "ChannelCombinedStatus_1_CH1_8"=40, "ChannelCombinedStatus_2_CH9_12"=41, "PlotData"=45, "PlotCommand"=46, "InternalData"=47, "KeepAlive"=234, "WakeUp"=250] ("commandID")
                    n116 = invoke class="PowerKvaserCom" method="SendPacket"(reference=w368, error in=w371, "priority"=w367, "commandID"=w365, "payload"=w366) -> (error out=w370:errorcluster, "SendPacket"=w369:bool)  [unwired: 1 in, 4 out]
                  }
                  frame "SW reset" {
                    w372 = u8 36 items=["ChannelStatus_1"=0, "ChannelControl"=2, "Current_CH1_4"=3, "Current_CH5_8"=4, "Current_CH9_12"=5, "Current_CH13_16"=6, "GetVinVout"=8, "Version_BoardType"=9, "SystemTemp"=10, "SystemParameter"=11, "ChannelParameter"=12, "GetTripEvent"=15, "LogFile"=18, "Configuration"=19, "ProductionData"=20, "BIT"=33, "DiscretePorts"=34, "SerialNumber"=36, "OffsetMeasurement"=37, "PartNumber"=39, "ChannelCombinedStatus_1_CH1_8"=40, "ChannelCombinedStatus_2_CH9_12"=41, "PlotData"=45, "PlotCommand"=46, "InternalData"=47, "KeepAlive"=234, "WakeUp"=250] ("commandID")
                    n117 = invoke class="PowerKvaserCom" method="SendPacket"(reference=w375, error in=w378, "priority"=w374, "commandID"=w372, "payload"=w373) -> (error out=w377:errorcluster, "SendPacket"=w376:bool)  [unwired: 1 in, 4 out]
                  }
                  frame "Get CH STS" {
                    w379 = u8 0 items=["ChannelStatus_1"=0, "ChannelControl"=2, "Current_CH1_4"=3, "Current_CH5_8"=4, "Current_CH9_12"=5, "Current_CH13_16"=6, "GetVinVout"=8, "Version_BoardType"=9, "SystemTemp"=10, "SystemParameter"=11, "ChannelParameter"=12, "GetTripEvent"=15, "LogFile"=18, "Configuration"=19, "ProductionData"=20, "BIT"=33, "DiscretePorts"=34, "SerialNumber"=36, "OffsetMeasurement"=37, "PartNumber"=39, "ChannelCombinedStatus_1_CH1_8"=40, "ChannelCombinedStatus_2_CH9_12"=41, "PlotData"=45, "PlotCommand"=46, "InternalData"=47, "KeepAlive"=234, "WakeUp"=250] ("commandID")
                    n118 = invoke class="PowerKvaserCom" method="SendPacket"(reference=w382, error in=w385, "priority"=w381, "commandID"=w379, "payload"=w380) -> (error out=w384:errorcluster, "SendPacket"=w383:bool)  [unwired: 1 in, 4 out]
                  }
                  frame "Get CH Current" {
                    n119 = case shown="1..4, Default" w386 {
                      tunnel: [w394 w395 w396 w397] -> w387
                      frame 1..4, Default {
                        w394 = u8 3 items=["ChannelStatus_1"=0, "ChannelControl"=2, "Current_CH1_4"=3, "Current_CH5_8"=4, "Current_CH9_12"=5, "Current_CH13_16"=6, "GetVinVout"=8, "Version_BoardType"=9, "SystemTemp"=10, "SystemParameter"=11, "ChannelParameter"=12, "GetTripEvent"=15, "LogFile"=18, "Configuration"=19, "ProductionData"=20, "BIT"=33, "DiscretePorts"=34, "SerialNumber"=36, "OffsetMeasurement"=37, "PartNumber"=39, "ChannelCombinedStatus_1_CH1_8"=40, "ChannelCombinedStatus_2_CH9_12"=41, "PlotData"=45, "PlotCommand"=46, "InternalData"=47, "KeepAlive"=234, "WakeUp"=250] ("commandID")
                      }
                      frame 5..8 {
                        w395 = u8 4 items=["ChannelStatus_1"=0, "ChannelControl"=2, "Current_CH1_4"=3, "Current_CH5_8"=4, "Current_CH9_12"=5, "Current_CH13_16"=6, "GetVinVout"=8, "Version_BoardType"=9, "SystemTemp"=10, "SystemParameter"=11, "ChannelParameter"=12, "GetTripEvent"=15, "LogFile"=18, "Configuration"=19, "ProductionData"=20, "BIT"=33, "DiscretePorts"=34, "SerialNumber"=36, "OffsetMeasurement"=37, "PartNumber"=39, "ChannelCombinedStatus_1_CH1_8"=40, "ChannelCombinedStatus_2_CH9_12"=41, "PlotData"=45, "PlotCommand"=46, "InternalData"=47, "KeepAlive"=234, "WakeUp"=250] ("commandID")
                      }
                      frame 9..12 {
                        w396 = u8 5 items=["ChannelStatus_1"=0, "ChannelControl"=2, "Current_CH1_4"=3, "Current_CH5_8"=4, "Current_CH9_12"=5, "Current_CH13_16"=6, "GetVinVout"=8, "Version_BoardType"=9, "SystemTemp"=10, "SystemParameter"=11, "ChannelParameter"=12, "GetTripEvent"=15, "LogFile"=18, "Configuration"=19, "ProductionData"=20, "BIT"=33, "DiscretePorts"=34, "SerialNumber"=36, "OffsetMeasurement"=37, "PartNumber"=39, "ChannelCombinedStatus_1_CH1_8"=40, "ChannelCombinedStatus_2_CH9_12"=41, "PlotData"=45, "PlotCommand"=46, "InternalData"=47, "KeepAlive"=234, "WakeUp"=250] ("commandID")
                      }
                      frame 13..16 {
                        w397 = u8 6 items=["ChannelStatus_1"=0, "ChannelControl"=2, "Current_CH1_4"=3, "Current_CH5_8"=4, "Current_CH9_12"=5, "Current_CH13_16"=6, "GetVinVout"=8, "Version_BoardType"=9, "SystemTemp"=10, "SystemParameter"=11, "ChannelParameter"=12, "GetTripEvent"=15, "LogFile"=18, "Configuration"=19, "ProductionData"=20, "BIT"=33, "DiscretePorts"=34, "SerialNumber"=36, "OffsetMeasurement"=37, "PartNumber"=39, "ChannelCombinedStatus_1_CH1_8"=40, "ChannelCombinedStatus_2_CH9_12"=41, "PlotData"=45, "PlotCommand"=46, "InternalData"=47, "KeepAlive"=234, "WakeUp"=250] ("commandID")
                      }
                    }
                    n120 = invoke class="PowerKvaserCom" method="SendPacket"(reference=w390, error in=w393, "priority"=w389, "commandID"=w387, "payload"=w388) -> (error out=w392:errorcluster, "SendPacket"=w391:bool)  [unwired: 1 in, 4 out]
                  }
                  frame "Get CH Voltage" {
                    w400 = u8 8 items=["ChannelStatus_1"=0, "ChannelControl"=2, "Current_CH1_4"=3, "Current_CH5_8"=4, "Current_CH9_12"=5, "Current_CH13_16"=6, "GetVinVout"=8, "Version_BoardType"=9, "SystemTemp"=10, "SystemParameter"=11, "ChannelParameter"=12, "GetTripEvent"=15, "LogFile"=18, "Configuration"=19, "ProductionData"=20, "BIT"=33, "DiscretePorts"=34, "SerialNumber"=36, "OffsetMeasurement"=37, "PartNumber"=39, "ChannelCombinedStatus_1_CH1_8"=40, "ChannelCombinedStatus_2_CH9_12"=41, "PlotData"=45, "PlotCommand"=46, "InternalData"=47, "KeepAlive"=234, "WakeUp"=250] ("commandID")
                    n121 = Build Array(w399) -> (w398:u8[])
                    n122 = invoke class="PowerKvaserCom" method="SendPacket"(reference=w402, error in=w405, "priority"=w401, "commandID"=w400, "payload"=w398) -> (error out=w404:errorcluster, "SendPacket"=w403:bool)  [unwired: 1 in, 4 out]
                  }
                  frame "CH Cnt" {
                    w426 = u8 2 items=["ChannelStatus_1"=0, "ChannelControl"=2, "Current_CH1_4"=3, "Current_CH5_8"=4, "Current_CH9_12"=5, "Current_CH13_16"=6, "GetVinVout"=8, "Version_BoardType"=9, "SystemTemp"=10, "SystemParameter"=11, "ChannelParameter"=12, "GetTripEvent"=15, "LogFile"=18, "Configuration"=19, "ProductionData"=20, "BIT"=33, "DiscretePorts"=34, "SerialNumber"=36, "OffsetMeasurement"=37, "PartNumber"=39, "ChannelCombinedStatus_1_CH1_8"=40, "ChannelCombinedStatus_2_CH9_12"=41, "PlotData"=45, "PlotCommand"=46, "InternalData"=47, "KeepAlive"=234, "WakeUp"=250] ("commandID")
                    n123 = Decrement(x=w415) -> (x-1=w425:u8)
                    n124 = local read "CH Cnt"() -> (w406:bool)
                    n125 = To Long Integer(number=w425) -> (32bit integer=w419:i32)
                    n126 = Number To Boolean Array(number=u16 0 ("element")) -> (Boolean array=w423:bool[])
                    n127 = Replace Array Subset(array=w423, new element=w406, index=w419) -> (w422:bool[])
                    n128 = Number To Boolean Array(number=u16 4095 ("mask")) -> (Boolean array=w420:bool[])
                    n129 = Boolean Array To Number(Boolean array=w422) -> (number=w421:u32)
                    n130 = To Unsigned Word Integer(number=w421) -> (unsigned 16bit integer=w413:u16)
                    n131 = Replace Array Subset(array=w420, new element=FALSE ("new element/subarray"), index=w419) -> (w424:bool[])
                    n132 = Split Number(x=w413) -> (hi(x)=w409:u8, lo(x)=w410:u8)
                    n133 = Boolean Array To Number(Boolean array=w424) -> (number=w414:u32)
                    n134 = To Unsigned Word Integer(number=w414) -> (unsigned 16bit integer=w411:u16)
                    n135 = Split Number(x=w411) -> (hi(x)=w407:u8, lo(x)=w408:u8)
                    n136 = Build Array(w410, w408, w409, w407) -> (w412:u8[])
                    n137 = invoke class="PowerKvaserCom" method="SendPacket"(reference=w428, error in=w431, "priority"=w427, "commandID"=w426, "payload"=w412) -> (error out=w430:errorcluster, "SendPacket"=w429:bool)  [unwired: 1 in, 4 out]
                  }
                  frame "Get Unit Name" {
                    n138 = invoke on="Unit name 8msg" class="PowerKvaserCom" method="AskSysUnitName"(reference=w435, error in=w434, "priority"=w433) -> (error out=w436:errorcluster, "AskSysUnitName"=w437:bool)  [unwired: 1 in, 2 out]
                    n139 = local write "unit_name"("" ("unit_name")) -> ()
                  }
                  frame "Get SN" {
                    n140 = invoke on="S/n 2msg" class="PowerKvaserCom" method="AskSerialNumber"(reference=w441, error in=w440, "priority"=w439) -> (error out=w443:errorcluster, "AskSerialNumber"=w442:bool)  [unwired: 1 in, 2 out]
                    n141 = local write "sn_l"("" ("sn_l")) -> ()
                  }
                  frame "CH Param" {
                    n142 = local read "CHParamNumber"() -> (w444:u8)
                    n143 = Array Size(array=w448) -> (size(s)=w447:i32)
                    n144 = invoke on="CH param" class="PowerKvaserCom" method="SendChannelParamPacket"(reference=w446, error in=w445, "priority"=w451, "systemParamNumber"=w444, "channelNum"=w450, "payload"=w448, "strInd"=w447) -> (error out=w449:errorcluster, "SendChannelParamPacket"=w452:bool)  [unwired: 1 in, 6 out]
                  }
                  frame "Sys Param" {
                    n145 = local read "systemParamNumber"() -> (w453:u8)
                    n146 = Array Size(array=w454) -> (size(s)=w455:i32)
                    n147 = invoke on="Sys param" class="PowerKvaserCom" method="SendSysParamPacket"(reference=w458, error in=w457, "priority"=w456, "systemParamNumber"=w453, "payload"=w454, "strInd"=w455) -> (error out=w460:errorcluster, "SendSysParamPacket"=w459:bool)  [unwired: 1 in, 5 out]
                  }
                  frame "Get CH Name" {
                    n148 = invoke on="CH name , 6cmd" class="PowerKvaserCom" method="AskChannelUnitName"(reference=w465, error in=w464, "priority"=w466, "channelNumber"=w461) -> (error out=w463:errorcluster, "AskChannelUnitName"=w462:bool)  [unwired: 1 in, 3 out]
                  }
                }
              }
              frame 2 {
                w477 = refnum<k24> refnum  # CANalystRef
                n149 = Variant To Data(error in=w476, type=w477, Variant=w478) -> (data=w472:refnum<k24>, error out=w475:errorcluster)
                n150 = case shown="\"Get SW ver\"" w467 {
                  tunnel: w475 -> [w485 w492 w499 w506 w513 w521 w533 w559 w562 w568 w572 w584 w592]
                  tunnel: [w484 w491 w498 w505 w512 w520 w532 w558 w564 w571 w576 w587 w591] -> w474
                  tunnel: [w483 w490 w497 w504 w511 w519 w531 w557 w565 w570 w579 w586 w590] -> w473
                  tunnel: w472 -> [w482 w489 w496 w503 w510 w518 w530 w556 w563 w569 w573 w585 w593]
                  tunnel: w471 -> [w481 w488 w495 w502 w509 w517 w529 w555 w561 w567 w578 w583 w594]
                  tunnel: w470 -> [w480 _ _ _ _ _ _ _ _ _ _ _ _]
                  tunnel: w469 -> [w479 w487 w494 w501 w508 w516 _ _ _ _ w575 w581 _]
                  tunnel: w468 -> [_ _ _ _ _ w514 w527 w542 _ _ w577 _ w589]
                  frame "Send", Default {
                    n151 = invoke class="PowerCanalystCom" method="SendPacket"(reference=w482, error in=w485, "priority"=w481, "commandID"=w480, "payload"=w479) -> (error out=w484:errorcluster, "SendPacket"=w483:bool)  [unwired: 1 in, 4 out]
                  }
                  frame "Get SW ver" {
                    w486 = u8 9 items=["ChannelStatus_1"=0, "ChannelControl"=2, "Current_CH1_4"=3, "Current_CH5_8"=4, "Current_CH9_12"=5, "Current_CH13_16"=6, "GetVinVout"=8, "Version_BoardType"=9, "SystemTemp"=10, "SystemParameter"=11, "ChannelParameter"=12, "GetTripEvent"=15, "LogFile"=18, "Configuration"=19, "ProductionData"=20, "BIT"=33, "DiscretePorts"=34, "SerialNumber"=36, "OffsetMeasurement"=37, "PartNumber"=39, "ChannelCombinedStatus_1_CH1_8"=40, "ChannelCombinedStatus_2_CH9_12"=41, "PlotData"=45, "PlotCommand"=46, "InternalData"=47, "KeepAlive"=234, "WakeUp"=250] ("commandID")
                    n152 = invoke class="PowerCanalystCom" method="SendPacket"(reference=w489, error in=w492, "priority"=w488, "commandID"=w486, "payload"=w487) -> (error out=w491:errorcluster, "SendPacket"=w490:bool)  [unwired: 1 in, 4 out]
                  }
                  frame "Get PN" {
                    w493 = u8 39 items=["ChannelStatus_1"=0, "ChannelControl"=2, "Current_CH1_4"=3, "Current_CH5_8"=4, "Current_CH9_12"=5, "Current_CH13_16"=6, "GetVinVout"=8, "Version_BoardType"=9, "SystemTemp"=10, "SystemParameter"=11, "ChannelParameter"=12, "GetTripEvent"=15, "LogFile"=18, "Configuration"=19, "ProductionData"=20, "BIT"=33, "DiscretePorts"=34, "SerialNumber"=36, "OffsetMeasurement"=37, "PartNumber"=39, "ChannelCombinedStatus_1_CH1_8"=40, "ChannelCombinedStatus_2_CH9_12"=41, "PlotData"=45, "PlotCommand"=46, "InternalData"=47, "KeepAlive"=234, "WakeUp"=250] ("commandID")
                    n153 = invoke class="PowerCanalystCom" method="SendPacket"(reference=w496, error in=w499, "priority"=w495, "commandID"=w493, "payload"=w494) -> (error out=w498:errorcluster, "SendPacket"=w497:bool)  [unwired: 1 in, 4 out]
                  }
                  frame "SW reset" {
                    w500 = u8 36 items=["ChannelStatus_1"=0, "ChannelControl"=2, "Current_CH1_4"=3, "Current_CH5_8"=4, "Current_CH9_12"=5, "Current_CH13_16"=6, "GetVinVout"=8, "Version_BoardType"=9, "SystemTemp"=10, "SystemParameter"=11, "ChannelParameter"=12, "GetTripEvent"=15, "LogFile"=18, "Configuration"=19, "ProductionData"=20, "BIT"=33, "DiscretePorts"=34, "SerialNumber"=36, "OffsetMeasurement"=37, "PartNumber"=39, "ChannelCombinedStatus_1_CH1_8"=40, "ChannelCombinedStatus_2_CH9_12"=41, "PlotData"=45, "PlotCommand"=46, "InternalData"=47, "KeepAlive"=234, "WakeUp"=250] ("commandID")
                    n154 = invoke class="PowerCanalystCom" method="SendPacket"(reference=w503, error in=w506, "priority"=w502, "commandID"=w500, "payload"=w501) -> (error out=w505:errorcluster, "SendPacket"=w504:bool)  [unwired: 1 in, 4 out]
                  }
                  frame "Get CH STS" {
                    w507 = u8 0 items=["ChannelStatus_1"=0, "ChannelControl"=2, "Current_CH1_4"=3, "Current_CH5_8"=4, "Current_CH9_12"=5, "Current_CH13_16"=6, "GetVinVout"=8, "Version_BoardType"=9, "SystemTemp"=10, "SystemParameter"=11, "ChannelParameter"=12, "GetTripEvent"=15, "LogFile"=18, "Configuration"=19, "ProductionData"=20, "BIT"=33, "DiscretePorts"=34, "SerialNumber"=36, "OffsetMeasurement"=37, "PartNumber"=39, "ChannelCombinedStatus_1_CH1_8"=40, "ChannelCombinedStatus_2_CH9_12"=41, "PlotData"=45, "PlotCommand"=46, "InternalData"=47, "KeepAlive"=234, "WakeUp"=250] ("commandID")
                    n155 = invoke class="PowerCanalystCom" method="SendPacket"(reference=w510, error in=w513, "priority"=w509, "commandID"=w507, "payload"=w508) -> (error out=w512:errorcluster, "SendPacket"=w511:bool)  [unwired: 1 in, 4 out]
                  }
                  frame "Get CH Current" {
                    n156 = case shown="1..4, Default" w514 {
                      tunnel: [w522 w523 w524 w525] -> w515
                      frame 1..4, Default {
                        w522 = u8 3 items=["ChannelStatus_1"=0, "ChannelControl"=2, "Current_CH1_4"=3, "Current_CH5_8"=4, "Current_CH9_12"=5, "Current_CH13_16"=6, "GetVinVout"=8, "Version_BoardType"=9, "SystemTemp"=10, "SystemParameter"=11, "ChannelParameter"=12, "GetTripEvent"=15, "LogFile"=18, "Configuration"=19, "ProductionData"=20, "BIT"=33, "DiscretePorts"=34, "SerialNumber"=36, "OffsetMeasurement"=37, "PartNumber"=39, "ChannelCombinedStatus_1_CH1_8"=40, "ChannelCombinedStatus_2_CH9_12"=41, "PlotData"=45, "PlotCommand"=46, "InternalData"=47, "KeepAlive"=234, "WakeUp"=250] ("commandID")
                      }
                      frame 5..8 {
                        w523 = u8 4 items=["ChannelStatus_1"=0, "ChannelControl"=2, "Current_CH1_4"=3, "Current_CH5_8"=4, "Current_CH9_12"=5, "Current_CH13_16"=6, "GetVinVout"=8, "Version_BoardType"=9, "SystemTemp"=10, "SystemParameter"=11, "ChannelParameter"=12, "GetTripEvent"=15, "LogFile"=18, "Configuration"=19, "ProductionData"=20, "BIT"=33, "DiscretePorts"=34, "SerialNumber"=36, "OffsetMeasurement"=37, "PartNumber"=39, "ChannelCombinedStatus_1_CH1_8"=40, "ChannelCombinedStatus_2_CH9_12"=41, "PlotData"=45, "PlotCommand"=46, "InternalData"=47, "KeepAlive"=234, "WakeUp"=250] ("commandID")
                      }
                      frame 9..12 {
                        w524 = u8 5 items=["ChannelStatus_1"=0, "ChannelControl"=2, "Current_CH1_4"=3, "Current_CH5_8"=4, "Current_CH9_12"=5, "Current_CH13_16"=6, "GetVinVout"=8, "Version_BoardType"=9, "SystemTemp"=10, "SystemParameter"=11, "ChannelParameter"=12, "GetTripEvent"=15, "LogFile"=18, "Configuration"=19, "ProductionData"=20, "BIT"=33, "DiscretePorts"=34, "SerialNumber"=36, "OffsetMeasurement"=37, "PartNumber"=39, "ChannelCombinedStatus_1_CH1_8"=40, "ChannelCombinedStatus_2_CH9_12"=41, "PlotData"=45, "PlotCommand"=46, "InternalData"=47, "KeepAlive"=234, "WakeUp"=250] ("commandID")
                      }
                      frame 13..16 {
                        w525 = u8 6 items=["ChannelStatus_1"=0, "ChannelControl"=2, "Current_CH1_4"=3, "Current_CH5_8"=4, "Current_CH9_12"=5, "Current_CH13_16"=6, "GetVinVout"=8, "Version_BoardType"=9, "SystemTemp"=10, "SystemParameter"=11, "ChannelParameter"=12, "GetTripEvent"=15, "LogFile"=18, "Configuration"=19, "ProductionData"=20, "BIT"=33, "DiscretePorts"=34, "SerialNumber"=36, "OffsetMeasurement"=37, "PartNumber"=39, "ChannelCombinedStatus_1_CH1_8"=40, "ChannelCombinedStatus_2_CH9_12"=41, "PlotData"=45, "PlotCommand"=46, "InternalData"=47, "KeepAlive"=234, "WakeUp"=250] ("commandID")
                      }
                    }
                    n157 = invoke class="PowerCanalystCom" method="SendPacket"(reference=w518, error in=w521, "priority"=w517, "commandID"=w515, "payload"=w516) -> (error out=w520:errorcluster, "SendPacket"=w519:bool)  [unwired: 1 in, 4 out]
                  }
                  frame "Get CH Voltage" {
                    w528 = u8 8 items=["ChannelStatus_1"=0, "ChannelControl"=2, "Current_CH1_4"=3, "Current_CH5_8"=4, "Current_CH9_12"=5, "Current_CH13_16"=6, "GetVinVout"=8, "Version_BoardType"=9, "SystemTemp"=10, "SystemParameter"=11, "ChannelParameter"=12, "GetTripEvent"=15, "LogFile"=18, "Configuration"=19, "ProductionData"=20, "BIT"=33, "DiscretePorts"=34, "SerialNumber"=36, "OffsetMeasurement"=37, "PartNumber"=39, "ChannelCombinedStatus_1_CH1_8"=40, "ChannelCombinedStatus_2_CH9_12"=41, "PlotData"=45, "PlotCommand"=46, "InternalData"=47, "KeepAlive"=234, "WakeUp"=250] ("commandID")
                    n158 = Build Array(w527) -> (w526:u8[])
                    n159 = invoke class="PowerCanalystCom" method="SendPacket"(reference=w530, error in=w533, "priority"=w529, "commandID"=w528, "payload"=w526) -> (error out=w532:errorcluster, "SendPacket"=w531:bool)  [unwired: 1 in, 4 out]
                  }
                  frame "CH Cnt" {
                    w554 = u8 2 items=["ChannelStatus_1"=0, "ChannelControl"=2, "Current_CH1_4"=3, "Current_CH5_8"=4, "Current_CH9_12"=5, "Current_CH13_16"=6, "GetVinVout"=8, "Version_BoardType"=9, "SystemTemp"=10, "SystemParameter"=11, "ChannelParameter"=12, "GetTripEvent"=15, "LogFile"=18, "Configuration"=19, "ProductionData"=20, "BIT"=33, "DiscretePorts"=34, "SerialNumber"=36, "OffsetMeasurement"=37, "PartNumber"=39, "ChannelCombinedStatus_1_CH1_8"=40, "ChannelCombinedStatus_2_CH9_12"=41, "PlotData"=45, "PlotCommand"=46, "InternalData"=47, "KeepAlive"=234, "WakeUp"=250] ("commandID")
                    n160 = Decrement(x=w542) -> (x-1=w552:u8)
                    n161 = To Long Integer(number=w552) -> (32bit integer=w546:i32)
                    n162 = Number To Boolean Array(number=u16 0 ("element")) -> (Boolean array=w550:bool[])
                    n163 = Replace Array Subset(array=w550, new element="CH Cnt", index=w546) -> (w549:bool[])
                    n164 = Number To Boolean Array(number=u16 4095 ("mask")) -> (Boolean array=w547:bool[])
                    n165 = Boolean Array To Number(Boolean array=w549) -> (number=w548:u32)
                    n166 = To Unsigned Word Integer(number=w548) -> (unsigned 16bit integer=w540:u16)
                    n167 = Replace Array Subset(array=w547, new element=FALSE ("new element/subarray"), index=w546) -> (w551:bool[])
                    n168 = Split Number(x=w540) -> (hi(x)=w536:u8, lo(x)=w537:u8)
                    n169 = Boolean Array To Number(Boolean array=w551) -> (number=w541:u32)
                    n170 = To Unsigned Word Integer(number=w541) -> (unsigned 16bit integer=w538:u16)
                    n171 = Split Number(x=w538) -> (hi(x)=w534:u8, lo(x)=w535:u8)
                    n172 = Build Array(w537, w535, w536, w534) -> (w539:u8[])
                    n173 = invoke class="PowerCanalystCom" method="SendPacket"(reference=w556, error in=w559, "priority"=w555, "commandID"=w554, "payload"=w539) -> (error out=w558:errorcluster, "SendPacket"=w557:bool)  [unwired: 1 in, 4 out]
                  }
                  frame "Get Unit Name" {
                    n174 = invoke on="Unit name 8msg" class="PowerCanalystCom" method="AskSysUnitName"(reference=w563, error in=w562, "priority"=w561) -> (error out=w564:errorcluster, "AskSysUnitName"=w565:bool)  [unwired: 1 in, 2 out]
                    n175 = local write "unit_name"("" ("unit_name")) -> ()
                  }
                  frame "Get SN" {
                    n176 = invoke on="S/n 2msg" class="PowerCanalystCom" method="AskSerialNumber"(reference=w569, error in=w568, "priority"=w567) -> (error out=w571:errorcluster, "AskSerialNumber"=w570:bool)  [unwired: 1 in, 2 out]
                    n177 = local write "sn_l"("" ("sn_l")) -> ()
                  }
                  frame "CH Param" {
                    n178 = Array Size(array=w575) -> (size(s)=w574:i32)
                    n179 = invoke on="CH param" class="PowerCanalystCom" method="SendChannelParamPacket"(reference=w573, error in=w572, "priority"=w578, "systemParamNumber"="CHParamNumber", "channelNum"=w577, "payload"=w575, "strInd"=w574) -> (error out=w576:errorcluster, "SendChannelParamPacket"=w579:bool)  [unwired: 1 in, 6 out]
                  }
                  frame "Sys Param" {
                    n180 = Array Size(array=w581) -> (size(s)=w582:i32)
                    n181 = invoke on="Sys param" class="PowerCanalystCom" method="SendSysParamPacket"(reference=w585, error in=w584, "priority"=w583, "systemParamNumber"="systemParamNumber", "payload"=w581, "strInd"=w582) -> (error out=w587:errorcluster, "SendSysParamPacket"=w586:bool)  [unwired: 1 in, 5 out]
                  }
                  frame "Get CH Name" {
                    n182 = invoke on="CH name , 6cmd" class="PowerCanalystCom" method="AskChannelUnitName"(reference=w593, error in=w592, "priority"=w594, "channelNumber"=w589) -> (error out=w591:errorcluster, "AskChannelUnitName"=w590:bool)  [unwired: 1 in, 3 out]
                  }
                }
              }
              frame 5 {
                w604 = refnum<k24> refnum  # UDP ref
                n183 = Variant To Data(error in=w605, type=w604, Variant=w606) -> (data=w596:refnum<k24>, error out=w595:errorcluster)
                n184 = case shown="\"Get SW ver\"" w603 {
                  tunnel: w595 -> [w613 w620 w627 w634 w641 w649 w661 w687 w690 w696 w701 w713 w720]
                  tunnel: [w612 w619 w626 w633 w640 w648 w660 w686 w692 w699 w705 w716 w719] -> w602
                  tunnel: [w611 w618 w625 w632 w639 w647 w659 w685 w693 w698 w708 w715 w718] -> w601
                  tunnel: w596 -> [w610 w617 w624 w631 w638 w646 w658 w684 w691 w697 w702 w714 w721]
                  tunnel: w600 -> [w609 w616 w623 w630 w637 w645 w657 w683 w689 w695 w707 w712 w722]
                  tunnel: w599 -> [w608 _ _ _ _ _ _ _ _ _ _ _ _]
                  tunnel: w598 -> [w607 w615 w622 _ w636 w644 _ _ _ _ w704 w710 _]
                  tunnel: w597 -> [_ _ _ _ _ w642 w655 w671 _ _ w706 _ w717]
                  frame "Send", Default {
                    n185 = invoke class="PowerUDPCom" method="SendPacket"(reference=w610, error in=w613, "priority"=w609, "commandID"=w608, "payload"=w607) -> (error out=w612:errorcluster, "SendPacket"=w611:bool)  [unwired: 1 in, 4 out]
                  }
                  frame "Get SW ver" {
                    w614 = u8 9 items=["ChannelStatus_1"=0, "ChannelControl"=2, "Current_CH1_4"=3, "Current_CH5_8"=4, "Current_CH9_12"=5, "Current_CH13_16"=6, "GetVinVout"=8, "Version_BoardType"=9, "SystemTemp"=10, "SystemParameter"=11, "ChannelParameter"=12, "GetTripEvent"=15, "LogFile"=18, "Configuration"=19, "ProductionData"=20, "BIT"=33, "DiscretePorts"=34, "SerialNumber"=36, "OffsetMeasurement"=37, "PartNumber"=39, "ChannelCombinedStatus_1_CH1_8"=40, "ChannelCombinedStatus_2_CH9_12"=41, "PlotData"=45, "PlotCommand"=46, "InternalData"=47, "KeepAlive"=234, "WakeUp"=250] ("commandID")
                    n186 = invoke class="PowerUDPCom" method="SendPacket"(reference=w617, error in=w620, "priority"=w616, "commandID"=w614, "payload"=w615) -> (error out=w619:errorcluster, "SendPacket"=w618:bool)  [unwired: 1 in, 4 out]
                  }
                  frame "Get PN" {
                    w621 = u8 39 items=["ChannelStatus_1"=0, "ChannelControl"=2, "Current_CH1_4"=3, "Current_CH5_8"=4, "Current_CH9_12"=5, "Current_CH13_16"=6, "GetVinVout"=8, "Version_BoardType"=9, "SystemTemp"=10, "SystemParameter"=11, "ChannelParameter"=12, "GetTripEvent"=15, "LogFile"=18, "Configuration"=19, "ProductionData"=20, "BIT"=33, "DiscretePorts"=34, "SerialNumber"=36, "OffsetMeasurement"=37, "PartNumber"=39, "ChannelCombinedStatus_1_CH1_8"=40, "ChannelCombinedStatus_2_CH9_12"=41, "PlotData"=45, "PlotCommand"=46, "InternalData"=47, "KeepAlive"=234, "WakeUp"=250] ("commandID")
                    n187 = invoke class="PowerUDPCom" method="SendPacket"(reference=w624, error in=w627, "priority"=w623, "commandID"=w621, "payload"=w622) -> (error out=w626:errorcluster, "SendPacket"=w625:bool)  [unwired: 1 in, 4 out]
                  }
                  frame "SW reset" {
                    w629 = u8 19 items=["ChannelStatus_1"=0, "ChannelControl"=2, "Current_CH1_4"=3, "Current_CH5_8"=4, "Current_CH9_12"=5, "Current_CH13_16"=6, "GetVinVout"=8, "Version_BoardType"=9, "SystemTemp"=10, "SystemParameter"=11, "ChannelParameter"=12, "GetTripEvent"=15, "LogFile"=18, "Configuration"=19, "ProductionData"=20, "BIT"=33, "DiscretePorts"=34, "SerialNumber"=36, "OffsetMeasurement"=37, "PartNumber"=39, "ChannelCombinedStatus_1_CH1_8"=40, "ChannelCombinedStatus_2_CH9_12"=41, "PlotData"=45, "PlotCommand"=46, "InternalData"=47, "KeepAlive"=234, "WakeUp"=250] ("commandID")
                    n188 = invoke class="PowerUDPCom" method="SendPacket"(reference=w631, error in=w634, "priority"=w630, "commandID"=w629, "payload"=u8[] [133, 162, 52, 25, 1]) -> (error out=w633:errorcluster, "SendPacket"=w632:bool)  [unwired: 1 in, 4 out]
                  }
                  frame "Get CH STS" {
                    w635 = u8 0 items=["ChannelStatus_1"=0, "ChannelControl"=2, "Current_CH1_4"=3, "Current_CH5_8"=4, "Current_CH9_12"=5, "Current_CH13_16"=6, "GetVinVout"=8, "Version_BoardType"=9, "SystemTemp"=10, "SystemParameter"=11, "ChannelParameter"=12, "GetTripEvent"=15, "LogFile"=18, "Configuration"=19, "ProductionData"=20, "BIT"=33, "DiscretePorts"=34, "SerialNumber"=36, "OffsetMeasurement"=37, "PartNumber"=39, "ChannelCombinedStatus_1_CH1_8"=40, "ChannelCombinedStatus_2_CH9_12"=41, "PlotData"=45, "PlotCommand"=46, "InternalData"=47, "KeepAlive"=234, "WakeUp"=250] ("commandID")
                    n189 = invoke class="PowerUDPCom" method="SendPacket"(reference=w638, error in=w641, "priority"=w637, "commandID"=w635, "payload"=w636) -> (error out=w640:errorcluster, "SendPacket"=w639:bool)  [unwired: 1 in, 4 out]
                  }
                  frame "Get CH Current" {
                    n190 = case shown="1..4, Default" w642 {
                      tunnel: [w650 w651 w652 w653] -> w643
                      frame 1..4, Default {
                        w650 = u8 3 items=["ChannelStatus_1"=0, "ChannelControl"=2, "Current_CH1_4"=3, "Current_CH5_8"=4, "Current_CH9_12"=5, "Current_CH13_16"=6, "GetVinVout"=8, "Version_BoardType"=9, "SystemTemp"=10, "SystemParameter"=11, "ChannelParameter"=12, "GetTripEvent"=15, "LogFile"=18, "Configuration"=19, "ProductionData"=20, "BIT"=33, "DiscretePorts"=34, "SerialNumber"=36, "OffsetMeasurement"=37, "PartNumber"=39, "ChannelCombinedStatus_1_CH1_8"=40, "ChannelCombinedStatus_2_CH9_12"=41, "PlotData"=45, "PlotCommand"=46, "InternalData"=47, "KeepAlive"=234, "WakeUp"=250] ("commandID")
                      }
                      frame 5..8 {
                        w651 = u8 4 items=["ChannelStatus_1"=0, "ChannelControl"=2, "Current_CH1_4"=3, "Current_CH5_8"=4, "Current_CH9_12"=5, "Current_CH13_16"=6, "GetVinVout"=8, "Version_BoardType"=9, "SystemTemp"=10, "SystemParameter"=11, "ChannelParameter"=12, "GetTripEvent"=15, "LogFile"=18, "Configuration"=19, "ProductionData"=20, "BIT"=33, "DiscretePorts"=34, "SerialNumber"=36, "OffsetMeasurement"=37, "PartNumber"=39, "ChannelCombinedStatus_1_CH1_8"=40, "ChannelCombinedStatus_2_CH9_12"=41, "PlotData"=45, "PlotCommand"=46, "InternalData"=47, "KeepAlive"=234, "WakeUp"=250] ("commandID")
                      }
                      frame 9..12 {
                        w652 = u8 5 items=["ChannelStatus_1"=0, "ChannelControl"=2, "Current_CH1_4"=3, "Current_CH5_8"=4, "Current_CH9_12"=5, "Current_CH13_16"=6, "GetVinVout"=8, "Version_BoardType"=9, "SystemTemp"=10, "SystemParameter"=11, "ChannelParameter"=12, "GetTripEvent"=15, "LogFile"=18, "Configuration"=19, "ProductionData"=20, "BIT"=33, "DiscretePorts"=34, "SerialNumber"=36, "OffsetMeasurement"=37, "PartNumber"=39, "ChannelCombinedStatus_1_CH1_8"=40, "ChannelCombinedStatus_2_CH9_12"=41, "PlotData"=45, "PlotCommand"=46, "InternalData"=47, "KeepAlive"=234, "WakeUp"=250] ("commandID")
                      }
                      frame 13..16 {
                        w653 = u8 6 items=["ChannelStatus_1"=0, "ChannelControl"=2, "Current_CH1_4"=3, "Current_CH5_8"=4, "Current_CH9_12"=5, "Current_CH13_16"=6, "GetVinVout"=8, "Version_BoardType"=9, "SystemTemp"=10, "SystemParameter"=11, "ChannelParameter"=12, "GetTripEvent"=15, "LogFile"=18, "Configuration"=19, "ProductionData"=20, "BIT"=33, "DiscretePorts"=34, "SerialNumber"=36, "OffsetMeasurement"=37, "PartNumber"=39, "ChannelCombinedStatus_1_CH1_8"=40, "ChannelCombinedStatus_2_CH9_12"=41, "PlotData"=45, "PlotCommand"=46, "InternalData"=47, "KeepAlive"=234, "WakeUp"=250] ("commandID")
                      }
                    }
                    n191 = invoke class="PowerUDPCom" method="SendPacket"(reference=w646, error in=w649, "priority"=w645, "commandID"=w643, "payload"=w644) -> (error out=w648:errorcluster, "SendPacket"=w647:bool)  [unwired: 1 in, 4 out]
                  }
                  frame "Get CH Voltage" {
                    w656 = u8 8 items=["ChannelStatus_1"=0, "ChannelControl"=2, "Current_CH1_4"=3, "Current_CH5_8"=4, "Current_CH9_12"=5, "Current_CH13_16"=6, "GetVinVout"=8, "Version_BoardType"=9, "SystemTemp"=10, "SystemParameter"=11, "ChannelParameter"=12, "GetTripEvent"=15, "LogFile"=18, "Configuration"=19, "ProductionData"=20, "BIT"=33, "DiscretePorts"=34, "SerialNumber"=36, "OffsetMeasurement"=37, "PartNumber"=39, "ChannelCombinedStatus_1_CH1_8"=40, "ChannelCombinedStatus_2_CH9_12"=41, "PlotData"=45, "PlotCommand"=46, "InternalData"=47, "KeepAlive"=234, "WakeUp"=250] ("commandID")
                    n192 = Build Array(w655) -> (w654:u8[])
                    n193 = invoke class="PowerUDPCom" method="SendPacket"(reference=w658, error in=w661, "priority"=w657, "commandID"=w656, "payload"=w654) -> (error out=w660:errorcluster, "SendPacket"=w659:bool)  [unwired: 1 in, 4 out]
                  }
                  frame "CH Cnt" {
                    w682 = u8 2 items=["ChannelStatus_1"=0, "ChannelControl"=2, "Current_CH1_4"=3, "Current_CH5_8"=4, "Current_CH9_12"=5, "Current_CH13_16"=6, "GetVinVout"=8, "Version_BoardType"=9, "SystemTemp"=10, "SystemParameter"=11, "ChannelParameter"=12, "GetTripEvent"=15, "LogFile"=18, "Configuration"=19, "ProductionData"=20, "BIT"=33, "DiscretePorts"=34, "SerialNumber"=36, "OffsetMeasurement"=37, "PartNumber"=39, "ChannelCombinedStatus_1_CH1_8"=40, "ChannelCombinedStatus_2_CH9_12"=41, "PlotData"=45, "PlotCommand"=46, "InternalData"=47, "KeepAlive"=234, "WakeUp"=250] ("commandID")
                    n194 = Decrement(x=w671) -> (x-1=w681:u8)
                    n195 = local read "CH Cnt"() -> (w662:bool)
                    n196 = To Long Integer(number=w681) -> (32bit integer=w675:i32)
                    n197 = Number To Boolean Array(number=u16 0 ("element")) -> (Boolean array=w679:bool[])
                    n198 = Replace Array Subset(array=w679, new element=w662, index=w675) -> (w678:bool[])
                    n199 = Number To Boolean Array(number=u16 4095 ("mask")) -> (Boolean array=w676:bool[])
                    n200 = Boolean Array To Number(Boolean array=w678) -> (number=w677:u32)
                    n201 = To Unsigned Word Integer(number=w677) -> (unsigned 16bit integer=w669:u16)
                    n202 = Replace Array Subset(array=w676, new element=FALSE ("new element/subarray"), index=w675) -> (w680:bool[])
                    n203 = Split Number(x=w669) -> (hi(x)=w665:u8, lo(x)=w666:u8)
                    n204 = Boolean Array To Number(Boolean array=w680) -> (number=w670:u32)
                    n205 = To Unsigned Word Integer(number=w670) -> (unsigned 16bit integer=w667:u16)
                    n206 = Split Number(x=w667) -> (hi(x)=w663:u8, lo(x)=w664:u8)
                    n207 = Build Array(w666, w664, w665, w663) -> (w668:u8[])
                    n208 = invoke class="PowerUDPCom" method="SendPacket"(reference=w684, error in=w687, "priority"=w683, "commandID"=w682, "payload"=w668) -> (error out=w686:errorcluster, "SendPacket"=w685:bool)  [unwired: 1 in, 4 out]
                  }
                  frame "Get Unit Name" {
                    n209 = invoke on="Unit name 8msg" class="PowerUDPCom" method="AskSysUnitName"(reference=w691, error in=w690, "priority"=w689) -> (error out=w692:errorcluster, "AskSysUnitName"=w693:bool)  [unwired: 1 in, 2 out]
                    n210 = local write "unit_name"("" ("unit_name")) -> ()
                  }
                  frame "Get SN" {
                    n211 = invoke on="S/n 2msg" class="PowerUDPCom" method="AskSerialNumber"(reference=w697, error in=w696, "priority"=w695) -> (error out=w699:errorcluster, "AskSerialNumber"=w698:bool)  [unwired: 1 in, 2 out]
                    n212 = local write "sn_l"("" ("sn_l")) -> ()
                  }
                  frame "CH Param" {
                    n213 = local read "CHParamNumber"() -> (w700:u8)
                    n214 = Array Size(array=w704) -> (size(s)=w703:i32)
                    n215 = invoke on="CH param" class="PowerUDPCom" method="SendChannelParamPacket"(reference=w702, error in=w701, "priority"=w707, "systemParamNumber"=w700, "channelNum"=w706, "payload"=w704, "strInd"=w703) -> (error out=w705:errorcluster, "SendChannelParamPacket"=w708:bool)  [unwired: 1 in, 6 out]
                  }
                  frame "Sys Param" {
                    n216 = local read "systemParamNumber"() -> (w709:u8)
                    n217 = Array Size(array=w710) -> (size(s)=w711:i32)
                    n218 = invoke on="Sys param" class="PowerUDPCom" method="SendSysParamPacket"(reference=w714, error in=w713, "priority"=w712, "systemParamNumber"=w709, "payload"=w710, "strInd"=w711) -> (error out=w716:errorcluster, "SendSysParamPacket"=w715:bool)  [unwired: 1 in, 5 out]
                  }
                  frame "Get CH Name" {
                    n219 = invoke on="CH name , 6cmd" class="PowerUDPCom" method="AskChannelUnitName"(reference=w721, error in=w720, "priority"=w722, "channelNumber"=w717) -> (error out=w719:errorcluster, "AskChannelUnitName"=w718:bool)  [unwired: 1 in, 3 out]
                  }
                }
              }
            }
          }
        }
        "SendOK" <- w193
      }
      event "COMType": Value Change {
        n220 = event-data() -> ()  [unwired: 1 in, 6 out]
        n221 = local read "COMType"() -> (w724:u16)
        n222 = case shown="7" w724 {
          tunnel: [enum32{"CAN", "Serial", "UDP"}."CAN" ("Com type") enum32{"CAN", "Serial", "UDP"}."UDP" ("Com type") enum32{"CAN", "Serial", "UDP"}."Serial" ("Com type") enum32{"CAN", "Serial", "UDP"}."CAN" ("Com type")] -> w723
          frame 2, Default {
          }
          frame 5 {
          }
          frame 6 {
          }
          frame 7 {
          }
        }
        n223 = local write "Com type"(w723) -> ()
      }
      event "Disonnect": Value Change {
        n224 = event-data() -> ()  [unwired: 1 in, 1 out]
        n225 = local read "CommIcon"() -> (w732:bool)
        n226 = local read "COMType"() -> (w731:u16)
        n227 = local read "COM"() -> (w730:variant)
        n228 = case shown="True" w732 {
          tunnel: w730 -> [_ w737]
          tunnel: w731 -> [_ w736]
          tunnel: errorcluster {"status"=FALSE, "code"=0, "source"=""} ("error out") -> [_ w735]
          frame False {
          }
          frame True {
            n229 = case shown="7" w736 {
              tunnel: w737 -> [w742 w749 w757 w763]
              tunnel: w735 -> [w744 w751 w758 w764]
              tunnel: [w739 w746 w753 w760] -> _
              tunnel: [w738 w745 w752 w759] -> w734
              frame 6, Default {
                w743 = refnum<k24> refnum  # SerialCOMRef
                n230 = Variant To Data(error in=w744, type=w743, Variant=w742) -> (data=w740:refnum<k24>, error out=w741:errorcluster)
                n231 = invoke on="Close com" class="PowerSerialCom" method="CloseCom"(reference=w740, error in=w741) -> (error out=w739:errorcluster, "CloseCom"=w738:bool)  [unwired: 1 in, 1 out]
              }
              frame 7 {
                w750 = refnum<k24> refnum  # KvaserRef
                n232 = Variant To Data(error in=w751, type=w750, Variant=w749) -> (data=w748:refnum<k24>, error out=w747:errorcluster)
                n233 = invoke on="Close com" class="PowerKvaserCom" method="CloseCom"(reference=w748, error in=w747) -> (error out=w746:errorcluster, "CloseCom"=w745:bool)  [unwired: 1 in, 1 out]
              }
              frame 5 {
                w756 = refnum<k24> refnum  # UDP ref
                n234 = Variant To Data(error in=w758, type=w756, Variant=w757) -> (data=w755:refnum<k24>, error out=w754:errorcluster)
                n235 = invoke on="Close com" class="PowerUDPCom" method="CloseCom"(reference=w755, error in=w754) -> (error out=w753:errorcluster, "CloseCom"=w752:bool)  [unwired: 1 in, 1 out]
              }
              frame 2 {
                w765 = refnum<k24> refnum  # CANalystRef
                n236 = Variant To Data(error in=w764, type=w765, Variant=w763) -> (data=w761:refnum<k24>, error out=w762:errorcluster)
                n237 = invoke on="Close com" class="PowerCanalystCom" method="CloseCom"(reference=w761, error in=w762) -> (error out=w760:errorcluster, "CloseCom"=w759:bool)  [unwired: 1 in, 1 out]
              }
            }
            n238 = Not(x=w734) -> (.not. x?=w733:bool)
            n239 = local write "CommIcon"(w733) -> ()
          }
        }
      }
      event "stop m": Value Change {
        n240 = event-data() -> ()  [unwired: 1 in, 6 out]
        n241 = flat-sequence {
          frame #0 {
            n242 = local write "stop Int"(FALSE ("stop Int")) -> ()
          }
          frame #1 {
            n243 = Wait (ms)(milliseconds to wait=u32 10) -> ()  [unwired: 1 out]
          }
        }
      }
    }
  }
  n244 = while {
    tunnel: w2 -> [w771]
    stop <- "stop Int" stop-if-true
    n245 = local read "CommIcon"() -> (w768:bool)
    n246 = case shown="True" w768 {
      tunnel: w771 -> [_ w773]
      frame False {
      }
      frame True {
        n247 = Get Queue Status(queue=w773) -> (error out=w772:errorcluster, # elements in queue=w774:i32)  [unwired: 1 in, 7 out]
        n248 = case shown="1, Default" w774 {
          tunnel: w773 -> [_ w781]
          tunnel: w772 -> [_ w780]
          frame 0 {
          }
          frame 1, Default {
            n249 = local read "Select CH #"() -> (w775:u8)
            n250 = Dequeue Element(queue=w781, error in (no error)=w780) -> (element=w779:T2)  [unwired: 4 out]
            n251 = Unbundle By Name(w779) -> ("ID"=w778:u32, "aDATA"=w777:u8[])  [unwired: 1 out]
            n252 = Decrement(x=w775) -> (x-1=w776:u8)
            n253 = case shown="9" w778 {
              tunnel: w777 -> [_ w786 w815 w862 w870 w895 w920 w945 w965 w980 w993 w1022]
              tunnel: w776 -> [_ _ w805 _ w864 w889 w914 w939 _ _ _ _]
              tunnel: w775 -> [_ _ w807 _ w865 w890 w915 w940 _ _ _ _]
              frame 256, Default {
              }
              frame 9 {
                w788 = "."
                n254 = Index Array(array=w786, index #1=0 ("index")) -> (element #1=w792:u8, element #2=w793:u8, element #3=w797:u8, element #4=w794:u8)  [unwired: 7 in, 4 out]
                n255 = Number To Decimal String(number=w792, width (-)=i16 2) -> (decimal integer string=w800:string)
                n256 = Number To Decimal String(number=w793, width (-)=i16 2) -> (decimal integer string=w799:string)
                n257 = Build Array(w794) -> (w795:u8[])
                n258 = Number To Decimal String(number=w797, width (-)=i16 2) -> (decimal integer string=w798:string)
                n259 = Byte Array To String(unsigned byte array=w795) -> (string=w796:string)
                n260 = Concatenate Strings(w798, w788, w799, w788, w800, w788, w796) -> (w783:string)
                "SW ver" <- w783
                n261 = local read "String"() -> (w785:string)
                n262 = call "dataDisplay.vi"("string data"=w783, "string in"=w785, "string type"="SW ver:") -> ("str out"=w784:string)  [unwired: 8 in]
                n263 = local write "String"(w784) -> ()
              }
              frame 0 {
                # "CH 1..10 status"
                n264 = Quotient & Remainder(x=w805, y=2) -> (x-y*floor(x/y)=w804:i32, floor(x/y)=w803:i32)
                n265 = Number To Decimal String(number=w807, width (-)=i16 1) -> (decimal integer string=w812:string)
                n266 = Multiply(x=w804, y=u8 4) -> (x*y=w802:i32)
                n267 = Index Array(array=w815, index=w803) -> (element=w816:u8)
                n268 = Add(x=w802, y=u8 2) -> (x+y=w801:i32)
                n269 = Number To Boolean Array "Trip"(number=w816) -> (Boolean array=w814:bool[])
                n270 = property on="TripType Enum" class="Enum (strict)"() -> ("Strings []"=w827:string[])  [unwired: 2 in, 2 out]
                n271 = Index Array(array=w814, index #1=w801) -> (element #1=w826:bool, element #2=w825:bool)  [unwired: 1 in]
                n272 = Index Array(array=w814, index #1=w802) -> (element #1=w823:bool, element #2=w824:bool)  [unwired: 1 in]
                n273 = Build Array(w826, w825) -> (w822:bool[])
                n274 = Build Array(w823, w824) -> (w821:bool[])
                n275 = Boolean Array To Number(Boolean array=w822) -> (number=w820:u32)
                n276 = Boolean Array To Number(Boolean array=w821) -> (number=w819:u32)
                n277 = property on="Status Enum" class="Enum (strict)"() -> ("Strings []"=w828:string[])  [unwired: 2 in, 2 out]
                n278 = To Unsigned Word Integer(number=w819) -> (unsigned 16bit integer=w829:u16)
                n279 = Index Array(array=w827, index=w829) -> (element=w809:string)
                n280 = To Unsigned Byte Integer(number=w820) -> (unsigned 8bit integer=w830:u8)
                n281 = Index Array(array=w828, index=w830) -> (element=w808:string)
                n282 = Concatenate Strings(w812, " status ", w808, "; Trip status ", w809) -> (w832:string)
                n283 = local read "String"() -> (w834:string)
                n284 = call "dataDisplay.vi"("string data"=w832, "string in"=w834, "string type"="CH") -> ("str out"=w833:string)  [unwired: 8 in]
                n285 = local write "String"(w833) -> ()
              }
              frame 8 {
                # "Vin/Vout"
                n286 = Index Array(array=w862, index #1=0 ("index")) -> (element #1=w855:u8, element #2=w854:u8, element #3=w853:u8, element #4=w852:u8, element #5=w847:u8)  [unwired: 4 in]
                n287 = Join Numbers(hi=w854, lo=w855) -> ((hi.lo)=w856:u16)
                n288 = Join Numbers(hi=w852, lo=w853) -> ((hi.lo)=w857:u16)
                n289 = To Double Precision Float(number=w857) -> (double precision float=w848:dbl)
                n290 = To Double Precision Float(number=w856) -> (double precision float=w850:dbl)
                n291 = Number To Decimal String(number=w847, width (-)=i16 2) -> (decimal integer string=w844:string)
                n292 = Divide(x=w848, y=10.0) -> (x/y=w838:dbl)
                n293 = Divide(x=w850, y=10.0) -> (x/y=w842:dbl)
                n294 = Number To Fractional String(number=w838, precision (6)=i16 2) -> (F-format string=w836:string)  [unwired: 2 in]
                n295 = Number To Fractional String(number=w842, precision (6)=i16 2) -> (F-format string=w840:string)  [unwired: 2 in]
                n296 = Concatenate Strings("CH" ("string"), w844, ": Vin " ("string"), w840, "[V] ,Vout " ("string"), w836, "[V]" ("string")) -> (w859:string)
                n297 = local read "String"() -> (w861:string)
                n298 = call "dataDisplay.vi"("string data"=w859, "string in"=w861, "string type"="Voltage ") -> ("str out"=w860:string)  [unwired: 8 in]
                n299 = local write "String"(w860) -> ()
              }
              frame 3 {
                # "3   Current CH1-CH4"
                # "Current"
                n300 = Quotient & Remainder(x=w864, y=u8 3) -> (x-y*floor(x/y)=w877:u8)  [unwired: 1 out]
                n301 = Multiply(x=w877, y=u8 2) -> (x*y=w876:u8)
                n302 = Index Array(array=w870, index #1=w876) -> (element #1=w874:u8, element #2=w875:u8)  [unwired: 1 in]
                n303 = Join Numbers(hi=w875, lo=w874) -> ((hi.lo)=w878:u16)
                n304 = Number To Decimal String(number=w865, width (-)=i16 2) -> (decimal integer string=w867:string)
                n305 = To Word Integer(number=w878) -> (16bit integer=w880:i16)
                n306 = To Double Precision Float(number=w880) -> (double precision float=w879:dbl)
                n307 = Divide(x=w879, y=10.0) -> (x/y=w869:dbl)
                n308 = Number To Fractional String(number=w869, precision (6)=i16 2) -> (F-format string=w881:string)  [unwired: 2 in]
                n309 = Concatenate Strings("CH" ("string"), w867, ": " ("string"), w881, "[A]" ("string")) -> (w886:string)
                n310 = local read "String"() -> (w888:string)
                n311 = call "dataDisplay.vi"("string data"=w886, "string in"=w888, "string type"="Current ") -> ("str out"=w887:string)  [unwired: 8 in]
                n312 = local write "String"(w887) -> ()
              }
              frame 4 {
                (unwired) u8 4 ("y")
                # "4  Current CH5-CH8"
                # "Current"
                n313 = Quotient & Remainder(x=w889, y=u8 3) -> (x-y*floor(x/y)=w902:u8)  [unwired: 1 out]
                n314 = Multiply(x=w902, y=u8 2) -> (x*y=w901:u8)
                n315 = Index Array(array=w895, index #1=w901) -> (element #1=w899:u8, element #2=w900:u8)  [unwired: 1 in]
                n316 = Join Numbers(hi=w900, lo=w899) -> ((hi.lo)=w903:u16)
                n317 = Number To Decimal String(number=w890, width (-)=i16 2) -> (decimal integer string=w892:string)
                n318 = To Word Integer(number=w903) -> (16bit integer=w905:i16)
                n319 = To Double Precision Float(number=w905) -> (double precision float=w904:dbl)
                n320 = Divide(x=w904, y=10.0) -> (x/y=w894:dbl)
                n321 = Number To Fractional String(number=w894, precision (6)=i16 2) -> (F-format string=w906:string)  [unwired: 2 in]
                n322 = Concatenate Strings("CH" ("string"), w892, ": " ("string"), w906, "[A]" ("string")) -> (w911:string)
                n323 = local read "String"() -> (w913:string)
                n324 = call "dataDisplay.vi"("string data"=w911, "string in"=w913, "string type"="Current ") -> ("str out"=w912:string)  [unwired: 8 in]
                n325 = local write "String"(w912) -> ()
              }
              frame 5 {
                (unwired) u8 4 ("y")
                # "5 Current CH9-CH12"
                # "Current"
                n326 = Quotient & Remainder(x=w914, y=u8 3) -> (x-y*floor(x/y)=w927:u8)  [unwired: 1 out]
                n327 = Multiply(x=w927, y=u8 2) -> (x*y=w926:u8)
                n328 = Index Array(array=w920, index #1=w926) -> (element #1=w924:u8, element #2=w925:u8)  [unwired: 1 in]
                n329 = Join Numbers(hi=w925, lo=w924) -> ((hi.lo)=w928:u16)
                n330 = Number To Decimal String(number=w915, width (-)=i16 2) -> (decimal integer string=w917:string)
                n331 = To Word Integer(number=w928) -> (16bit integer=w930:i16)
                n332 = To Double Precision Float(number=w930) -> (double precision float=w929:dbl)
                n333 = Divide(x=w929, y=10.0) -> (x/y=w919:dbl)
                n334 = Number To Fractional String(number=w919, precision (6)=i16 2) -> (F-format string=w931:string)  [unwired: 2 in]
                n335 = Concatenate Strings("CH" ("string"), w917, ": " ("string"), w931, "[A]" ("string")) -> (w936:string)
                n336 = local read "String"() -> (w938:string)
                n337 = call "dataDisplay.vi"("string data"=w936, "string in"=w938, "string type"="Current ") -> ("str out"=w937:string)  [unwired: 8 in]
                n338 = local write "String"(w937) -> ()
              }
              frame 6 {
                (unwired) u8 4 ("y")
                # "6 Current CH13-CH16"
                # "Current"
                n339 = Quotient & Remainder(x=w939, y=u8 3) -> (x-y*floor(x/y)=w952:u8)  [unwired: 1 out]
                n340 = Multiply(x=w952, y=u8 2) -> (x*y=w951:u8)
                n341 = Index Array(array=w945, index #1=w951) -> (element #1=w949:u8, element #2=w950:u8)  [unwired: 1 in]
                n342 = Join Numbers(hi=w950, lo=w949) -> ((hi.lo)=w953:u16)
                n343 = Number To Decimal String(number=w940, width (-)=i16 2) -> (decimal integer string=w942:string)
                n344 = To Word Integer(number=w953) -> (16bit integer=w955:i16)
                n345 = To Double Precision Float(number=w955) -> (double precision float=w954:dbl)
                n346 = Divide(x=w954, y=10.0) -> (x/y=w944:dbl)
                n347 = Number To Fractional String(number=w944, precision (6)=i16 2) -> (F-format string=w956:string)  [unwired: 2 in]
                n348 = Concatenate Strings("CH" ("string"), w942, ": " ("string"), w956, "[A]" ("string")) -> (w961:string)
                n349 = local read "String"() -> (w963:string)
                n350 = call "dataDisplay.vi"("string data"=w961, "string in"=w963, "string type"="Current ") -> ("str out"=w962:string)  [unwired: 8 in]
                n351 = local write "String"(w962) -> ()
              }
              frame 39 {
                # "PN"
                n352 = Delete From Array(array=w965, length=4, index=4) -> (deleted portion=w971:u8[])  [unwired: 1 out]
                n353 = Delete From Array(array=w965, length=4, index=0) -> (deleted portion=w970:u8[])  [unwired: 1 out]
                n354 = Byte Array To String(unsigned byte array=w971) -> (string=w972:string)
                n355 = Byte Array To String(unsigned byte array=w970) -> (string=w973:string)
                n356 = Concatenate Strings(w972, w973) -> (w964:string)
                "PN ver" <- w964
                n357 = local read "String"() -> (w976:string)
                n358 = call "dataDisplay.vi"("string data"=w964, "string in"=w976, "string type"="PN ver:") -> ("str out"=w975:string)  [unwired: 8 in]
                n359 = local write "String"(w975) -> ()
              }
              frame 36 {
                # "PN"
                # "S/N"
                n360 = Index Array(array=w980, index=7) -> (element=w978:u8)
                n361 = Delete From Array(array=w980, length=6, index=0) -> (deleted portion=w983:u8[])  [unwired: 1 out]
                n362 = Byte Array To String(unsigned byte array=w983) -> (string=w977:string)
                n363 = case shown="6" w978 {
                  tunnel: w977 -> [w984 w985]
                  frame 0, Default {
                    "sn_l" <- w984
                  }
                  frame 6 {
                    n364 = local read "sn_l"() -> (w986:string)
                    n365 = local read "String"() -> (w990:string)
                    n366 = Concatenate Strings(w986, w985) -> (w987:string)
                    n367 = call "dataDisplay.vi"("string data"=w987, "string in"=w990, "string type"="Unit S/N :") -> ("str out"=w989:string)  [unwired: 8 in]
                    n368 = local write "String"(w989) -> ()
                  }
                }
              }
              frame 11 {
                # "System param"
                n369 = Index Array(array=w993, index=6) -> (element=w991:u8)
                n370 = case shown="9" w991 {
                  tunnel: w993 -> [_ w997]
                  frame 0, Default {
                  }
                  frame 9 {
                    # "Unit name"
                    n371 = Index Array(array=w997, index=7) -> (element=w995:u8)
                    n372 = Delete From Array(array=w997, length=6, index=0) -> (deleted portion=w1000:u8[])  [unwired: 1 out]
                    n373 = Byte Array To String(unsigned byte array=w1000) -> (string=w994:string)
                    n374 = case shown="0, Default" w995 {
                      selector: w995 -> [_ w1002 _]
                      tunnel: w994 -> [w1001 w1004 w1007]
                      frame 0, Default {
                        "unit_name" <- w1001
                      }
                      frame 6, 12 {
                        n375 = local read "unit_name"() -> (w1006:string)
                        n376 = Replace Substring(2:6 ("length (len. of substring)"), 3:w1002, 4:w1004, 5:w1006) -> (1:w1005:string)  [unwired: 1 out]
                        n377 = local write "unit_name"(w1005) -> ()
                      }
                      frame 18 {
                        n378 = local read "unit_name"() -> (w1008:string)
                        n379 = local read "String"() -> (w1012:string)
                        n380 = Concatenate Strings(w1008, w1007) -> (w1009:string)
                        n381 = call "dataDisplay.vi"("string data"=w1009, "string in"=w1012, "string type"="Unit Name:") -> ("str out"=w1011:string)  [unwired: 8 in]
                        n382 = local write "String"(w1011) -> ()
                      }
                    }
                  }
                }
              }
              frame 12 {
                # "CH param"
                n383 = Index Array(array=w1022, index #1=6 ("index")) -> (element #1=w1019:u8, element #2=w1016:u8)  [unwired: 1 in]
                n384 = And(x=w1019, y=u8 63) -> (x .and. y?=w1017:u8)
                n385 = Logical Shift(y=i8 -2, x=w1016) -> (x << y=w1014:u8)
                n386 = Number To Decimal String(number=w1014, width (-)=i16 2) -> (decimal integer string=w1013:string)
                n387 = case shown="5" w1017 {
                  tunnel: w1022 -> [_ w1040]
                  tunnel: w1013 -> [_ w1023]
                  frame 0, Default {
                  }
                  frame 5 {
                    # "Unit name"
                    n388 = Index Array(array=w1040, index #1=6 ("index")) -> (element #1=w1026:u8, element #2=w1025:u8)  [unwired: 1 in]
                    n389 = Number To Boolean Array(number=w1025) -> (Boolean array=w1031:bool[])
                    n390 = Number To Boolean Array(number=w1026) -> (Boolean array=w1030:bool[])
                    n391 = Index Array(array=w1030, index #1=5 ("index")) -> (element #1=w1032:bool, element #2=w1034:bool, element #3=w1035:bool)  [unwired: 2 in]
                    n392 = Index Array(array=w1031, index #1=0 ("index")) -> (element #1=w1036:bool, element #2=w1037:bool)  [unwired: 1 in]
                    n393 = Build Array(w1032, w1034, w1035, w1036, w1037) -> (w1033:bool[])
                    n394 = Delete From Array(array=w1040, length=6, index=0) -> (deleted portion=w1042:u8[])  [unwired: 1 out]
                    n395 = Byte Array To String(unsigned byte array=w1042) -> (string=w1038:string)
                    n396 = Boolean Array To Number(Boolean array=w1033) -> (number=w1027:u32)
                    n397 = case shown="12" w1027 {
                      selector: w1027 -> [_ w1044 _]
                      tunnel: w1038 -> [w1043 w1046 w1054]
                      tunnel: w1023 -> [_ _ w1050]
                      frame 0, Default {
                        "ch_name" <- w1043
                      }
                      frame 6, 12 {
                        n398 = local read "ch_name"() -> (w1048:string)
                        n399 = Replace Substring(2:6 ("length (len. of substring)"), 3:w1044, 4:w1046, 5:w1048) -> (1:w1047:string)  [unwired: 1 out]
                        n400 = local write "ch_name"(w1047) -> ()
                      }
                      frame 18 {
                        n401 = local read "ch_name"() -> (w1053:string)
                        n402 = Concatenate Strings(w1053, w1054) -> (w1055:string)
                        n403 = local read "String"() -> (w1057:string)
                        n404 = Concatenate Strings("CH " ("string type"), w1050, " Name:" ("string type")) -> (w1052:string)
                        n405 = call "dataDisplay.vi"("string data"=w1055, "string in"=w1057, "string type"=w1052) -> ("str out"=w1056:string)  [unwired: 8 in]
                        n406 = local write "String"(w1056) -> ()
                      }
                    }
                  }
                }
              }
            }
          }
        }
      }
    }
    n407 = Wait (ms)(milliseconds to wait=u32 5) -> ()  [unwired: 1 out]
  }
  n408 = flat-sequence {
    tunnel: w5 -> [w1062]
    tunnel: w1 -> [w1063]
    frame #0 {
      w1058 = FALSE ("stop Int")
      n409 = local read "COMType"() -> (w1061:u16)
      n410 = local read "COM"() -> (w1059:variant)
      n411 = local read "CommIcon"() -> (w1064:bool)
      n412 = local write "stop Int"(w1058) -> ()
      n413 = case shown="True" w1064 {
        tunnel: w1059 -> [_ w1093]
        tunnel: w1061 -> [_ w1092]
        tunnel: w1062 -> [w1089 w1091]
        tunnel: [w1089 w1090] -> w1060
        tunnel: w1058 -> [_ _]
        frame False {
        }
        frame True {
          n414 = case shown="6, Default" w1092 {
            tunnel: w1093 -> [w1098 w1105 w1113 w1119]
            tunnel: w1091 -> [w1100 w1107 w1114 w1120]
            tunnel: [w1095 w1102 w1109 w1116] -> w1090
            tunnel: [w1094 w1101 w1108 w1115] -> _
            frame 6, Default {
              w1099 = refnum<k24> refnum  # SerialCOMRef
              n415 = Variant To Data(error in=w1100, type=w1099, Variant=w1098) -> (data=w1096:refnum<k24>, error out=w1097:errorcluster)
              n416 = invoke on="Close com" class="PowerSerialCom" method="CloseCom"(reference=w1096, error in=w1097) -> (error out=w1095:errorcluster, "CloseCom"=w1094:bool)  [unwired: 1 in, 1 out]
            }
            frame 7 {
              w1106 = refnum<k24> refnum  # KvaserRef
              n417 = Variant To Data(error in=w1107, type=w1106, Variant=w1105) -> (data=w1104:refnum<k24>, error out=w1103:errorcluster)
              n418 = invoke on="Close com" class="PowerKvaserCom" method="CloseCom"(reference=w1104, error in=w1103) -> (error out=w1102:errorcluster, "CloseCom"=w1101:bool)  [unwired: 1 in, 1 out]
            }
            frame 5 {
              w1112 = refnum<k24> refnum  # UDP ref
              n419 = Variant To Data(error in=w1114, type=w1112, Variant=w1113) -> (data=w1111:refnum<k24>, error out=w1110:errorcluster)
              n420 = invoke on="Close com" class="PowerUDPCom" method="CloseCom"(reference=w1111, error in=w1110) -> (error out=w1109:errorcluster, "CloseCom"=w1108:bool)  [unwired: 1 in, 1 out]
            }
            frame 2 {
              w1121 = refnum<k24> refnum  # CANalystRef
              n421 = Variant To Data(error in=w1120, type=w1121, Variant=w1119) -> (data=w1117:refnum<k24>, error out=w1118:errorcluster)
              n422 = invoke on="Close com" class="PowerCanalystCom" method="CloseCom"(reference=w1117, error in=w1118) -> (error out=w1116:errorcluster, "CloseCom"=w1115:bool)  [unwired: 1 in, 1 out]
            }
          }
        }
      }
      n423 = Release Queue(queue=w1063, error in (no error)=w1062) -> ()  [unwired: 1 in, 3 out]
      n424 = case shown="6, Default" w1061 {
        tunnel: w1059 -> [w1068 w1074 w1081 w1086]
        tunnel: w1060 -> [w1070 w1076 w1082 w1087]
        tunnel: [w1065 w1072 w1079 w1083] -> _
        frame 6, Default {
          w1069 = refnum<k24> refnum  # SerialCOMRef
          n425 = Variant To Data(error in=w1070, type=w1069, Variant=w1068) -> (data=w1066:refnum<k24>, error out=w1067:errorcluster)
          n426 = Close Reference(reference=w1066, error in (no error)=w1067) -> (error out=w1065:errorcluster)
        }
        frame 7 {
          w1075 = refnum<k24> refnum  # KvaserRef
          n427 = Variant To Data(error in=w1076, type=w1075, Variant=w1074) -> (data=w1073:refnum<k24>, error out=w1071:errorcluster)
          n428 = Close Reference(reference=w1073, error in (no error)=w1071) -> (error out=w1072:errorcluster)
        }
        frame 5 {
          w1077 = refnum<k24> refnum  # UDP ref
          n429 = Variant To Data(error in=w1082, type=w1077, Variant=w1081) -> (data=w1080:refnum<k24>, error out=w1078:errorcluster)
          n430 = Close Reference(reference=w1080, error in (no error)=w1078) -> (error out=w1079:errorcluster)
        }
        frame 2 {
          w1088 = refnum<k24> refnum  # CANalystRef
          n431 = Variant To Data(error in=w1087, type=w1088, Variant=w1086) -> (data=w1085:refnum<k24>, error out=w1084:errorcluster)
          n432 = Close Reference(reference=w1085, error in (no error)=w1084) -> (error out=w1083:errorcluster)
        }
      }
    }
  }
